vi "GetStatus.vi"(8 "error in (no error)":errorcluster, 11 "S4ACS_GUI in":refnum<class "S4GUI.lvclass">) -> (0 "error out":errorcluster, 1 "output cluster":T2={"Trigger Mode Status"="", "String output"="", "Instrument Status"={"WPROT pos"=0.0, "WPSEL pos"=0.0, "GMIR pos"=0.0, "GFOC pos"=0.0, "CALW pos"=0.0, "ASEL pos"=0.0, "connection"=FALSE}, "Sync Box State"=0, "Trigger General Status"="", "Instrument States"={"WPSEL State"=0, "WPROT State"=0, "CALW State"=0, "ASEL State"=0, "GMIR State"=0, "GFOC State"=0}, "Instrument Pos Names"={"WPROT posname"="", "WPSEL posname"="", "CALW posname"="", "ASEL posname"=""}, "ChannelA_Status"={"Current exp"=0.0, "Frames done"=0, "LastFileImage"="", "CamStatus"="", "Run state"=0, "connection"=FALSE, "Cooler ON/OFF"=0, "Currently temperature"=20, "Temperature Status"=""}, "WPROT seq"=0, "ChannelB_Status"={"Current exp"=0.0, "Frames done"=0, "LastFileImage"="", "CamStatus"="", "Run state"=0, "connection"=FALSE, "Cooler ON/OFF"=0, "Currently temperature"=20, "Temperature Status"=""}, "ChannelC_Status"={"Current exp"=0.0, "Frames done"=0, "LastFileImage"="", "CamStatus"="", "Run state"=0, "connection"=FALSE, "Cooler ON/OFF"=0, "Currently temperature"=20, "Temperature Status"=""}, "ChannelD_Status"={"Current exp"=0.0, "Frames done"=0, "LastFileImage"="", "CamStatus"="", "Run state"=0, "connection"=FALSE, "Cooler ON/OFF"=0, "Currently temperature"=20, "Temperature Status"=""}, "ChannelA_CCD"={"ACQUISITION_MODE"=1, "TRIGGER_MODE"=0, "READ_MODE"=4, "PREAMP"=0, "READOUT_RATE"=0, "VERTICAL_SHIFT_SPEED"=3, "EM_MODE"=0, "EM_GAIN"=2, "SHUTTER_MODE"=2, "SHUTTER_TTL"=0, "SHUTTER_OPENNING_TIME"=50, "SHUTTER_CLOSING_TIME"=50, "VBIN"=1, "HBIN"=1, "INITIAL_LINE"=1, "INITIAL_COLUMN"=1, "FINAL_LINE"=1024, "FINAL_COLUMN"=1024, "FRAME_TRANSFER"=FALSE, "VERTICAL_CLOCK_VOLTAGE"=0, "AD_CHANNEL"=0}, "ChannelB_CCD "={"ACQUISITION_MODE"=1, "TRIGGER_MODE"=0, "READ_MODE"=4, "PREAMP"=0, "READOUT_RATE"=0, "VERTICAL_SHIFT_SPEED"=3, "EM_MODE"=0, "EM_GAIN"=2, "SHUTTER_MODE"=2, "SHUTTER_TTL"=0, "SHUTTER_OPENNING_TIME"=50, "SHUTTER_CLOSING_TIME"=50, "VBIN"=1, "HBIN"=1, "INITIAL_LINE"=1, "INITIAL_COLUMN"=1, "FINAL_LINE"=1024, "FINAL_COLUMN"=1024, "FRAME_TRANSFER"=FALSE, "VERTICAL_CLOCK_VOLTAGE"=0, "AD_CHANNEL"=0}, "ChannelC_CCD"={"ACQUISITION_MODE"=1, "TRIGGER_MODE"=0, "READ_MODE"=4, "PREAMP"=0, "READOUT_RATE"=0, "VERTICAL_SHIFT_SPEED"=3, "EM_MODE"=0, "EM_GAIN"=2, "SHUTTER_MODE"=2, "SHUTTER_TTL"=0, "SHUTTER_OPENNING_TIME"=50, "SHUTTER_CLOSING_TIME"=50, "VBIN"=1, "HBIN"=1, "INITIAL_LINE"=1, "INITIAL_COLUMN"=1, "FINAL_LINE"=1024, "FINAL_COLUMN"=1024, "FRAME_TRANSFER"=FALSE, "VERTICAL_CLOCK_VOLTAGE"=0, "AD_CHANNEL"=0}, "ChannelD_CCD"={"ACQUISITION_MODE"=1, "TRIGGER_MODE"=0, "READ_MODE"=4, "PREAMP"=0, "READOUT_RATE"=0, "VERTICAL_SHIFT_SPEED"=3, "EM_MODE"=0, "EM_GAIN"=2, "SHUTTER_MODE"=2, "SHUTTER_TTL"=0, "SHUTTER_OPENNING_TIME"=50, "SHUTTER_CLOSING_TIME"=50, "VBIN"=1, "HBIN"=1, "INITIAL_LINE"=1, "INITIAL_COLUMN"=1, "FINAL_LINE"=1024, "FINAL_COLUMN"=1024, "FRAME_TRANSFER"=FALSE, "VERTICAL_CLOCK_VOLTAGE"=0, "AD_CHANNEL"=0}, "CHA_Checked Params"={"ACQUISITION_MODE"=FALSE, "TRIGGER_MODE"=FALSE, "READ_MODE"=FALSE, "PREAMP"=FALSE, "READOUT_RATE"=FALSE, "VERTICAL_SHIFT_SPEED"=FALSE, "EM_MODE"=FALSE, "EM_GAIN"=FALSE, "SHUTTER_MODE"=FALSE, "SHUTTER_TTL"=FALSE, "SHUTTER_OPENING_TIME"=FALSE, "SHUTTER_CLOSING_TIME"=FALSE, "VBIN"=FALSE, "HBIN"=FALSE, "INITIAL_LINE"=FALSE, "INITIAL_COLUMN"=FALSE, "FINAL_LINE"=FALSE, "FINAL_COLUMN"=FALSE, "FRAME_TRANSFER"=FALSE, "VERTICAL_CLOCK_VOLTAGE"=FALSE, "AD_CHANNEL"=FALSE}, "CHB_Checked Params"={"ACQUISITION_MODE"=FALSE, "TRIGGER_MODE"=FALSE, "READ_MODE"=FALSE, "PREAMP"=FALSE, "READOUT_RATE"=FALSE, "VERTICAL_SHIFT_SPEED"=FALSE, "EM_MODE"=FALSE, "EM_GAIN"=FALSE, "SHUTTER_MODE"=FALSE, "SHUTTER_TTL"=FALSE, "SHUTTER_OPENING_TIME"=FALSE, "SHUTTER_CLOSING_TIME"=FALSE, "VBIN"=FALSE, "HBIN"=FALSE, "INITIAL_LINE"=FALSE, "INITIAL_COLUMN"=FALSE, "FINAL_LINE"=FALSE, "FINAL_COLUMN"=FALSE, "FRAME_TRANSFER"=FALSE, "VERTICAL_CLOCK_VOLTAGE"=FALSE, "AD_CHANNEL"=FALSE}, "CHC_Checked Params"={"ACQUISITION_MODE"=FALSE, "TRIGGER_MODE"=FALSE, "READ_MODE"=FALSE, "PREAMP"=FALSE, "READOUT_RATE"=FALSE, "VERTICAL_SHIFT_SPEED"=FALSE, "EM_MODE"=FALSE, "EM_GAIN"=FALSE, "SHUTTER_MODE"=FALSE, "SHUTTER_TTL"=FALSE, "SHUTTER_OPENING_TIME"=FALSE, "SHUTTER_CLOSING_TIME"=FALSE, "VBIN"=FALSE, "HBIN"=FALSE, "INITIAL_LINE"=FALSE, "INITIAL_COLUMN"=FALSE, "FINAL_LINE"=FALSE, "FINAL_COLUMN"=FALSE, "FRAME_TRANSFER"=FALSE, "VERTICAL_CLOCK_VOLTAGE"=FALSE, "AD_CHANNEL"=FALSE}, "CHD_Checked Params"={"ACQUISITION_MODE"=FALSE, "TRIGGER_MODE"=FALSE, "READ_MODE"=FALSE, "PREAMP"=FALSE, "READOUT_RATE"=FALSE, "VERTICAL_SHIFT_SPEED"=FALSE, "EM_MODE"=FALSE, "EM_GAIN"=FALSE, "SHUTTER_MODE"=FALSE, "SHUTTER_TTL"=FALSE, "SHUTTER_OPENING_TIME"=FALSE, "SHUTTER_CLOSING_TIME"=FALSE, "VBIN"=FALSE, "HBIN"=FALSE, "INITIAL_LINE"=FALSE, "INITIAL_COLUMN"=FALSE, "FINAL_LINE"=FALSE, "FINAL_COLUMN"=FALSE, "FRAME_TRANSFER"=FALSE, "VERTICAL_CLOCK_VOLTAGE"=FALSE, "AD_CHANNEL"=FALSE}, "Trigger_connection"=FALSE, "TCSPD_connection"=FALSE} {"ChannelD_CCD"."VERTICAL_CLOCK_VOLTAGE" items=["Normal", "+1", "+2", "+3", "+4"]; "ChannelD_CCD"."SHUTTER_TTL" items=["TTL Low", "TTl High"]; "ChannelD_CCD"."SHUTTER_MODE" items=["Fully Auto", "OPEN", "CLOSED"]; "ChannelD_CCD"."EM_MODE" items=["Electron Multiplying", "Conventional"]; "ChannelD_CCD"."VERTICAL_SHIFT_SPEED" items=["0.6", "1.13", "2.2", "4.33"]; "ChannelD_CCD"."READOUT_RATE" items=["1 MHz", "0.1 MHz", "10 MHz", "20 MHz", "30 MHz"]; "ChannelD_CCD"."PREAMP" items=["Gain 1", "Gain 2"]; "ChannelD_CCD"."READ_MODE" items=["Full Vertical Binning", "Multi-Track", "Random-track", "Single-Track", "Image"]; "ChannelD_CCD"."TRIGGER_MODE" items=["Internal", "External", "N/A", "N/A", "N/A", "N/A", "External Start"]; "ChannelD_CCD"."ACQUISITION_MODE" items=["None", "Single", "Accumulate", "Kinetics", "Fast Kinetics"]; "ChannelC_CCD"."VERTICAL_CLOCK_VOLTAGE" items=["Normal", "+1", "+2", "+3", "+4"]; "ChannelC_CCD"."SHUTTER_TTL" items=["TTL Low", "TTl High"]; "ChannelC_CCD"."SHUTTER_MODE" items=["Fully Auto", "OPEN", "CLOSED"]; "ChannelC_CCD"."EM_MODE" items=["Electron Multiplying", "Conventional"]; "ChannelC_CCD"."VERTICAL_SHIFT_SPEED" items=["0.6", "1.13", "2.2", "4.33"]; "ChannelC_CCD"."READOUT_RATE" items=["1 MHz", "0 .1 MHz", "10 MHz", "20 MHz", "30 MHz"]; "ChannelC_CCD"."PREAMP" items=["Gain 1", "Gain 2"]; "ChannelC_CCD"."READ_MODE" items=["Full Vertical Binning", "Multi-Track", "Random-track", "Single-Track", "Image"]; "ChannelC_CCD"."TRIGGER_MODE" items=["Internal", "External", "N/A", "N/A", "N/A", "N/A", "External Start"]; "ChannelC_CCD"."ACQUISITION_MODE" items=["None", "Single", "Accumulate", "Kinetics", "Fast Kinetics"]; "ChannelB_CCD"."VERTICAL_CLOCK_VOLTAGE" items=["Normal", "+1", "+2", "+3", "+4"]; "ChannelB_CCD"."SHUTTER_TTL" items=["TTL Low", "TTl High"]; "ChannelB_CCD"."SHUTTER_MODE" items=["Fully Auto", "OPEN", "CLOSED"]; "ChannelB_CCD"."EM_MODE" items=["Electron Multiplying", "Conventional"]; "ChannelB_CCD"."VERTICAL_SHIFT_SPEED" items=["0.6", "1.13", "2.2", "4.33"]; "ChannelB_CCD"."READOUT_RATE" items=["1 MHz", "0.1 MHz", "10 MHz", "20 MHz", "30 MHz"]; "ChannelB_CCD"."PREAMP" items=["Gain 1", "Gain 2"]; "ChannelB_CCD"."READ_MODE" items=["Full Vertical Binning", "Multi-Track", "Random-track", "Single-Track", "Image"]; "ChannelB_CCD"."TRIGGER_MODE" items=["Internal", "External", "N/A", "N/A", "N/A", "N/A", "External Start"]; "ChannelB_CCD"."ACQUISITION_MODE" items=["None", "Single", "Accumulate", "Kinetics", "Fast Kinetics"]; "ChannelA_CCD"."VERTICAL_CLOCK_VOLTAGE" items=["Normal", "+1", "+2", "+3", "+4"]; "ChannelA_CCD"."SHUTTER_TTL" items=["TTL Low", "TTl High"]; "ChannelA_CCD"."SHUTTER_MODE" items=["Fully Auto", "OPEN", "CLOSED"]; "ChannelA_CCD"."EM_MODE" items=["Electron Multiplying", "Conventional"]; "ChannelA_CCD"."VERTICAL_SHIFT_SPEED" items=["0.6", "1.13", "2.2", "4.33"]; "ChannelA_CCD"."READOUT_RATE" items=["1 MHz", "0.1 MHz", "10 MHz", "20 MHz", "30 MHz"]; "ChannelA_CCD"."PREAMP" items=["Gain 1", "Gain 2"]; "ChannelA_CCD"."READ_MODE" items=["Full Vertical Binning", "Multi-Track", "Random-track", "Single-Track", "Image"]; "ChannelA_CCD"."TRIGGER_MODE" items=["Internal", "External", "N/A", "N/A", "N/A", "N/A", "External Start"]; "ChannelA_CCD"."ACQUISITION_MODE" items=["None", "Single", "Accumulate", "Kinetics", "Fast Kinetics"]; "ChannelD_Status"."Currently temperature" min=0 max=0; "ChannelD_Status"."Cooler ON/OFF" items=["Cooler OFF", "Cooler ON"]; "ChannelC_Status"."Currently temperature" min=0 max=0; "ChannelC_Status"."Cooler ON/OFF" items=["Cooler OFF", "Cooler ON"]; "ChannelB_Status"."Currently temperature" min=0 max=0; "ChannelB_Status"."Cooler ON/OFF" items=["Cooler OFF", "Cooler ON"]; "ChannelA_Status"."Currently temperature" min=0 max=0; "ChannelA_Status"."Cooler ON/OFF" items=["Cooler OFF", "Cooler ON"]}, 2 "Cluster Disable":T1, 3 "S4ACS_GUI out":refnum<class "S4GUI.lvclass">)   [LabVIEW 2018, in "S4GUI.lvclass"]
uses:
  S4GUI.lvclass
  S4GUI.lvclass/S4GUI.ctl
  Server/Server.lvclass/Server.ctl
  Instrument/Instrument.lvclass/Instrument.ctl
  Device/Optics/Optics.lvclass/Optics.ctl
  Interface/Interface.lvclass/Interface.ctl
  TCS/TCS.lvclass
  C:/Users/observer/Desktop/Sparc4GUI/SPARC4_GUI/Server/Server.lvclass
  SyncBox/Sync Box.lvclass
  Device/Optics/Opt_Selector/Opt_Selector.lvclass
  C:/Users/observer/Desktop/Sparc4GUI/SPARC4_GUI/Device/Optics/Optics.lvclass
  Device/Optics/Opt_Continuous/Opt_Continuous.lvclass
  Instrument/Instrument.lvclass
  Acquisition/Acquisition.lvclass
  Channel/Channel.lvclass
  Interface/Interface.lvclass
  Trigger/Trigger.lvclass
  Device/Optics/Optics.lvclass
  Server/Server.lvclass
panel:
  in  "Cluster":T3={"Trigger Mode Status"="", "String output"="", "Instrument Status"={"WPROT pos"=0.0, "WPSEL pos"=0.0, "GMIR pos"=0.0, "GFOC pos"=0.0, "CALW pos"=0.0, "ASEL pos"=0.0, "connection"=FALSE}, "Sync Box State"=0, "Trigger General Status"="", "Instrument States"={"WPSEL State"=0, "WPROT State"=0, "CALW State"=0, "ASEL State"=0, "GMIR State"=0, "GFOC State"=0}, "Instrument Pos Names"={"WPROT posname"="", "WPSEL posname"="", "CALW posname"="", "ASEL posname"=""}, "ChannelA_Status"={"Current exp"=0.0, "Frames done"=0, "LastFileImage"="", "CamStatus"="", "Run state"=0, "connection"=FALSE, "Cooler ON/OFF"=0, "Currently temperature"=20, "Temperature Status"=""}, "WPROT seq"=0, "ChannelB_Status"={"Current exp"=0.0, "Frames done"=0, "LastFileImage"="", "CamStatus"="", "Run state"=0, "connection"=FALSE, "Cooler ON/OFF"=0, "Currently temperature"=20, "Temperature Status"=""}, "ChannelC_Status"={"Current exp"=0.0, "Frames done"=0, "LastFileImage"="", "CamStatus"="", "Run state"=0, "connection"=FALSE, "Cooler ON/OFF"=0, "Currently temperature"=20, "Temperature Status"=""}, "ChannelD_Status"={"Current exp"=0.0, "Frames done"=0, "LastFileImage"="", "CamStatus"="", "Run state"=0, "connection"=FALSE, "Cooler ON/OFF"=0, "Currently temperature"=20, "Temperature Status"=""}, "ChannelA_CCD"={"ACQUISITION_MODE"=1, "TRIGGER_MODE"=0, "READ_MODE"=4, "PREAMP"=0, "READOUT_RATE"=0, "VERTICAL_SHIFT_SPEED"=3, "EM_MODE"=0, "EM_GAIN"=2, "SHUTTER_MODE"=2, "SHUTTER_TTL"=0, "SHUTTER_OPENNING_TIME"=50, "SHUTTER_CLOSING_TIME"=50, "VBIN"=1, "HBIN"=1, "INITIAL_LINE"=1, "INITIAL_COLUMN"=1, "FINAL_LINE"=1024, "FINAL_COLUMN"=1024, "FRAME_TRANSFER"=FALSE, "VERTICAL_CLOCK_VOLTAGE"=0, "AD_CHANNEL"=0}, "ChannelB_CCD"={"ACQUISITION_MODE"=1, "TRIGGER_MODE"=0, "READ_MODE"=4, "PREAMP"=0, "READOUT_RATE"=0, "VERTICAL_SHIFT_SPEED"=3, "EM_MODE"=0, "EM_GAIN"=2, "SHUTTER_MODE"=2, "SHUTTER_TTL"=0, "SHUTTER_OPENNING_TIME"=50, "SHUTTER_CLOSING_TIME"=50, "VBIN"=1, "HBIN"=1, "INITIAL_LINE"=1, "INITIAL_COLUMN"=1, "FINAL_LINE"=1024, "FINAL_COLUMN"=1024, "FRAME_TRANSFER"=FALSE, "VERTICAL_CLOCK_VOLTAGE"=0, "AD_CHANNEL"=0}, "ChannelC_CCD"={"ACQUISITION_MODE"=1, "TRIGGER_MODE"=0, "READ_MODE"=4, "PREAMP"=0, "READOUT_RATE"=0, "VERTICAL_SHIFT_SPEED"=3, "EM_MODE"=0, "EM_GAIN"=2, "SHUTTER_MODE"=2, "SHUTTER_TTL"=0, "SHUTTER_OPENNING_TIME"=50, "SHUTTER_CLOSING_TIME"=50, "VBIN"=1, "HBIN"=1, "INITIAL_LINE"=1, "INITIAL_COLUMN"=1, "FINAL_LINE"=1024, "FINAL_COLUMN"=1024, "FRAME_TRANSFER"=FALSE, "VERTICAL_CLOCK_VOLTAGE"=0, "AD_CHANNEL"=0}, "ChannelD_CCD"={"ACQUISITION_MODE"=1, "TRIGGER_MODE"=0, "READ_MODE"=4, "PREAMP"=0, "READOUT_RATE"=0, "VERTICAL_SHIFT_SPEED"=3, "EM_MODE"=0, "EM_GAIN"=2, "SHUTTER_MODE"=2, "SHUTTER_TTL"=0, "SHUTTER_OPENNING_TIME"=50, "SHUTTER_CLOSING_TIME"=50, "VBIN"=1, "HBIN"=1, "INITIAL_LINE"=1, "INITIAL_COLUMN"=1, "FINAL_LINE"=1024, "FINAL_COLUMN"=1024, "FRAME_TRANSFER"=FALSE, "VERTICAL_CLOCK_VOLTAGE"=0, "AD_CHANNEL"=0}, "CHA_Checked Params"={"ACQUISITION_MODE"=FALSE, "TRIGGER_MODE"=FALSE, "READ_MODE"=FALSE, "PREAMP"=FALSE, "READOUT_RATE"=FALSE, "VERTICAL_SHIFT_SPEED"=FALSE, "EM_MODE"=FALSE, "EM_GAIN"=FALSE, "SHUTTER_MODE"=FALSE, "SHUTTER_TTL"=FALSE, "SHUTTER_OPENING_TIME"=FALSE, "SHUTTER_CLOSING_TIME"=FALSE, "VBIN"=FALSE, "HBIN"=FALSE, "INITIAL_LINE"=FALSE, "INITIAL_COLUMN"=FALSE, "FINAL_LINE"=FALSE, "FINAL_COLUMN"=FALSE, "FRAME_TRANSFER"=FALSE, "VERTICAL_CLOCK_VOLTAGE"=FALSE, "AD_CHANNEL"=FALSE}, "CHB_Checked Params"={"ACQUISITION_MODE"=FALSE, "TRIGGER_MODE"=FALSE, "READ_MODE"=FALSE, "PREAMP"=FALSE, "READOUT_RATE"=FALSE, "VERTICAL_SHIFT_SPEED"=FALSE, "EM_MODE"=FALSE, "EM_GAIN"=FALSE, "SHUTTER_MODE"=FALSE, "SHUTTER_TTL"=FALSE, "SHUTTER_OPENING_TIME"=FALSE, "SHUTTER_CLOSING_TIME"=FALSE, "VBIN"=FALSE, "HBIN"=FALSE, "INITIAL_LINE"=FALSE, "INITIAL_COLUMN"=FALSE, "FINAL_LINE"=FALSE, "FINAL_COLUMN"=FALSE, "FRAME_TRANSFER"=FALSE, "VERTICAL_CLOCK_VOLTAGE"=FALSE, "AD_CHANNEL"=FALSE}, "CHC_Checked Params"={"ACQUISITION_MODE"=FALSE, "TRIGGER_MODE"=FALSE, "READ_MODE"=FALSE, "PREAMP"=FALSE, "READOUT_RATE"=FALSE, "VERTICAL_SHIFT_SPEED"=FALSE, "EM_MODE"=FALSE, "EM_GAIN"=FALSE, "SHUTTER_MODE"=FALSE, "SHUTTER_TTL"=FALSE, "SHUTTER_OPENING_TIME"=FALSE, "SHUTTER_CLOSING_TIME"=FALSE, "VBIN"=FALSE, "HBIN"=FALSE, "INITIAL_LINE"=FALSE, "INITIAL_COLUMN"=FALSE, "FINAL_LINE"=FALSE, "FINAL_COLUMN"=FALSE, "FRAME_TRANSFER"=FALSE, "VERTICAL_CLOCK_VOLTAGE"=FALSE, "AD_CHANNEL"=FALSE}, "CHD_Checked Params"={"ACQUISITION_MODE"=FALSE, "TRIGGER_MODE"=FALSE, "READ_MODE"=FALSE, "PREAMP"=FALSE, "READOUT_RATE"=FALSE, "VERTICAL_SHIFT_SPEED"=FALSE, "EM_MODE"=FALSE, "EM_GAIN"=FALSE, "SHUTTER_MODE"=FALSE, "SHUTTER_TTL"=FALSE, "SHUTTER_OPENING_TIME"=FALSE, "SHUTTER_CLOSING_TIME"=FALSE, "VBIN"=FALSE, "HBIN"=FALSE, "INITIAL_LINE"=FALSE, "INITIAL_COLUMN"=FALSE, "FINAL_LINE"=FALSE, "FINAL_COLUMN"=FALSE, "FRAME_TRANSFER"=FALSE, "VERTICAL_CLOCK_VOLTAGE"=FALSE, "AD_CHANNEL"=FALSE}, "Trigger_connection"=FALSE, "TCSPD_connection"=FALSE} {"ChannelD_CCD"."VERTICAL_CLOCK_VOLTAGE" items=["Normal", "+1", "+2", "+3", "+4"]; "ChannelD_CCD"."SHUTTER_TTL" items=["TTL Low", "TTl High"]; "ChannelD_CCD"."SHUTTER_MODE" items=["Fully Auto", "OPEN", "CLOSED"]; "ChannelD_CCD"."EM_MODE" items=["Electron Multiplying", "Conventional"]; "ChannelD_CCD"."VERTICAL_SHIFT_SPEED" items=["0.6", "1.13", "2.2", "4.33"]; "ChannelD_CCD"."READOUT_RATE" items=["1 MHz", "0.1 MHz", "10 MHz", "20 MHz", "30 MHz"]; "ChannelD_CCD"."PREAMP" items=["Gain 1", "Gain 2"]; "ChannelD_CCD"."READ_MODE" items=["Full Vertical Binning", "Multi-Track", "Random-track", "Single-Track", "Image"]; "ChannelD_CCD"."TRIGGER_MODE" items=["Internal", "External", "N/A", "N/A", "N/A", "N/A", "External Start"]; "ChannelD_CCD"."ACQUISITION_MODE" items=["None", "Single", "Accumulate", "Kinetics", "Fast Kinetics"]; "ChannelC_CCD"."VERTICAL_CLOCK_VOLTAGE" items=["Normal", "+1", "+2", "+3", "+4"]; "ChannelC_CCD"."SHUTTER_TTL" items=["TTL Low", "TTl High"]; "ChannelC_CCD"."SHUTTER_MODE" items=["Fully Auto", "OPEN", "CLOSED"]; "ChannelC_CCD"."EM_MODE" items=["Electron Multiplying", "Conventional"]; "ChannelC_CCD"."VERTICAL_SHIFT_SPEED" items=["0.6", "1.13", "2.2", "4.33"]; "ChannelC_CCD"."READOUT_RATE" items=["1 MHz", "0.1 MHz", "10 MHz", "20 MHz", "30 MHz"]; "ChannelC_CCD"."PREAMP" items=["Gain 1", "Gain 2"]; "ChannelC_CCD"."READ_MODE" items=["Full Vertical Binning", "Multi-Track", "Random-track", "Single-Track", "Image"]; "ChannelC_CCD"."TRIGGER_MODE" items=["Internal", "External", "N/A", "N/A", "N/A", "N/A", "External Start"]; "ChannelC_CCD"."ACQUISITION_MODE" items=["None", "Single", "Accumulate", "Kinetics", "Fast Kinetics"]; "ChannelB_CCD"."VERTICAL_CLOCK_VOLTAGE" items=["Normal", "+1", "+2", "+3", "+4"]; "ChannelB_CCD"."SHUTTER_TTL" items=["TTL Low", "TTl High"]; "ChannelB_CCD"."SHUTTER_MODE" items=["Fully Auto", "OPEN", "CLOSED"]; "ChannelB_CCD"."EM_MODE" items=["Electron Multiplying", "Conventional"]; "ChannelB_CCD"."VERTICAL_SHIFT_SPEED" items=["0.6", "1.13", "2.2", "4.33"]; "ChannelB_CCD"."READOUT_RATE" items=["1 MHz", "0.1 MHz", "10 MHz", "20 MHz", "30 MHz"]; "ChannelB_CCD"."PREAMP" items=["Gain 1", "Gain 2"]; "ChannelB_CCD"."READ_MODE" items=["Full Vertical Binning", "Multi-Track", "Random-track", "Single-Track", "Image"]; "ChannelB_CCD"."TRIGGER_MODE" items=["Internal", "External", "N/A", "N/A", "N/A", "N/A", "External Start"]; "ChannelB_CCD"."ACQUISITION_MODE" items=["None", "Single", "Accumulate", "Kinetics", "Fast Kinetics"]; "ChannelA_CCD"."VERTICAL_CLOCK_VOLTAGE" items=["Normal", "+1", "+2", "+3", "+4"]; "ChannelA_CCD"."SHUTTER_TTL" items=["TTL Low", "TTl High"]; "ChannelA_CCD"."SHUTTER_MODE" items=["Fully Auto", "OPEN", "CLOSED"]; "ChannelA_CCD"."EM_MODE" items=["Electron Multiplying", "Conventional"]; "ChannelA_CCD"."VERTICAL_SHIFT_SPEED" items=["0.6", "1.13", "2.2", "4.33"]; "ChannelA_CCD"."READOUT_RATE" items=["1 MHz", "0.1 MHz", "10 MHz", "20 MHz", "30 MHz"]; "ChannelA_CCD"."PREAMP" items=["Gain 1", "Gain 2"]; "ChannelA_CCD"."READ_MODE" items=["Full Vertical Binning", "Multi-Track", "Random-track", "Single-Track", "Image"]; "ChannelA_CCD"."TRIGGER_MODE" items=["Internal", "External", "N/A", "N/A", "N/A", "N/A", "External Start"]; "ChannelA_CCD"."ACQUISITION_MODE" items=["None", "Single", "Accumulate", "Kinetics", "Fast Kinetics"]; "ChannelD_Status"."Currently temperature" min=0 max=0; "ChannelD_Status"."Cooler ON/OFF" items=["Cooler OFF", "Cooler ON"]; "ChannelC_Status"."Currently temperature" min=0 max=0; "ChannelC_Status"."Cooler ON/OFF" items=["Cooler OFF", "Cooler ON"]; "ChannelB_Status"."Currently temperature" min=0 max=0; "ChannelB_Status"."Cooler ON/OFF" items=["Cooler OFF", "Cooler ON"]; "ChannelA_Status"."Currently temperature" min=0 max=0; "ChannelA_Status"."Cooler ON/OFF" items=["Cooler OFF", "Cooler ON"]}
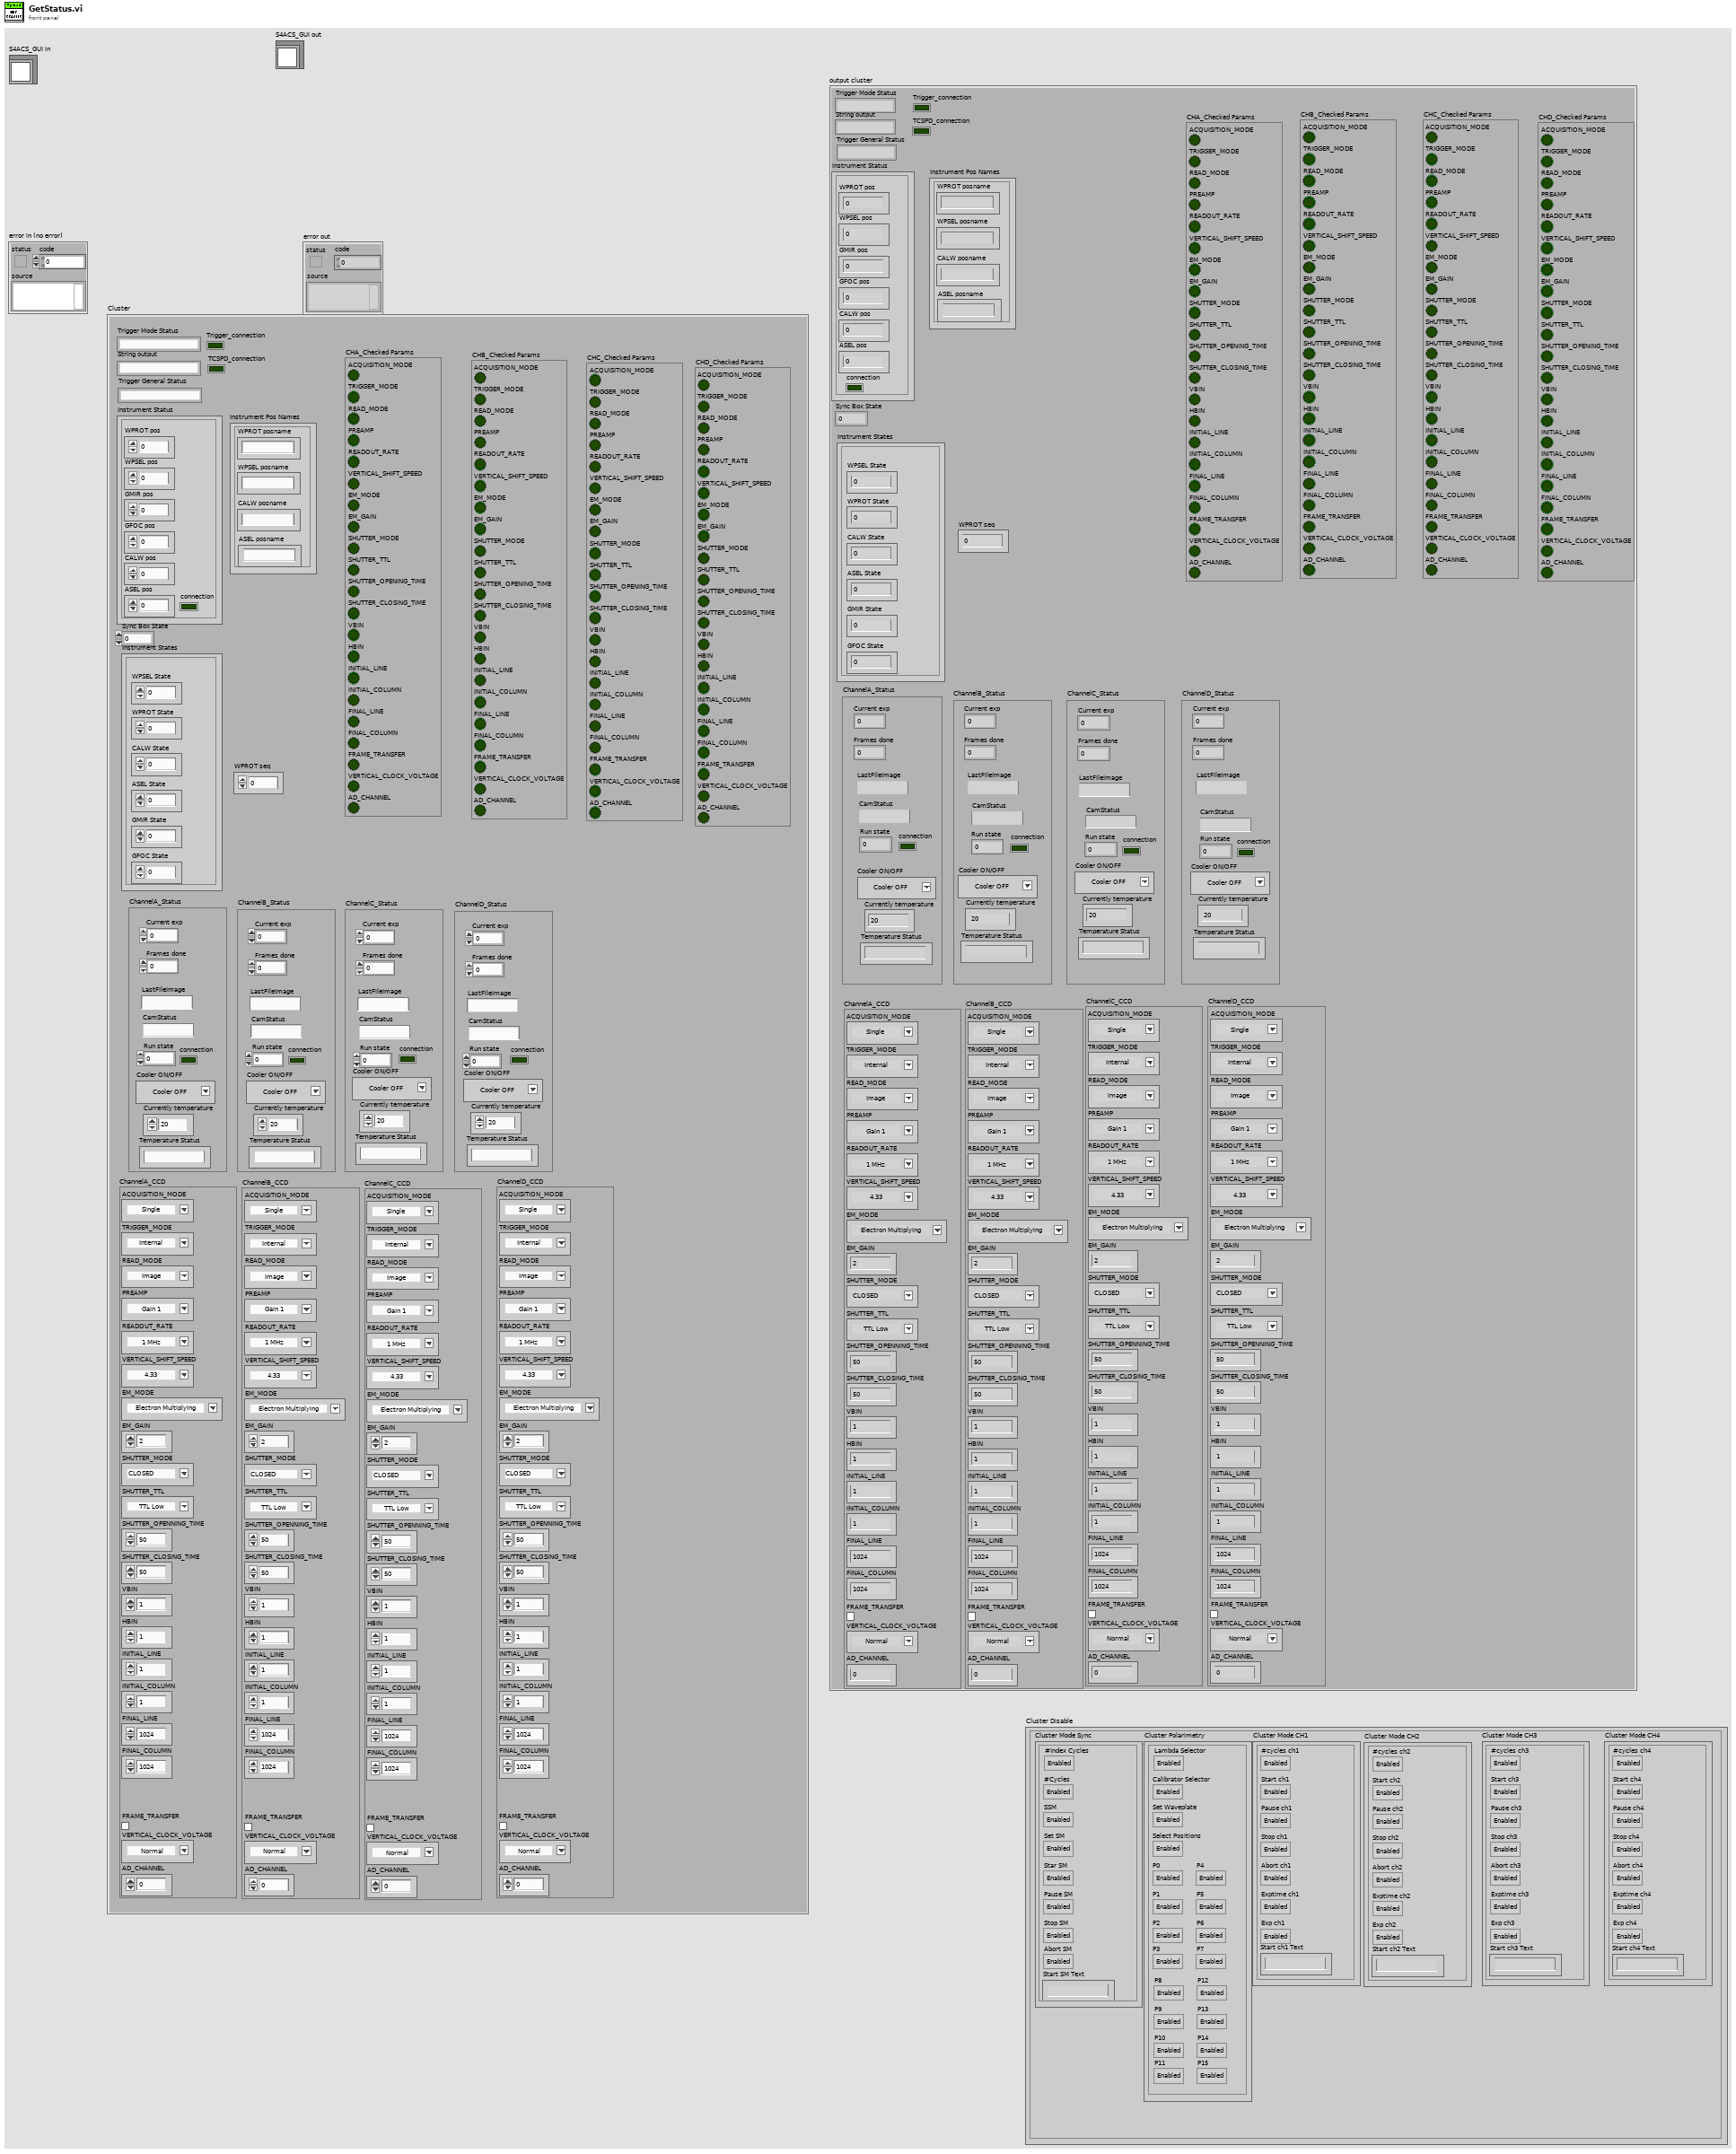
[diagram p1: front panel]
types:
  T1 = cluster{"Cluster Mode Sync":cluster{"#Index Cycles":enum8{"Enabled", "Disabled", "Disabled and Grayed Out"}, "#Cycles":enum8{"Enabled", "Disabled", "Disabled and Grayed Out"}, "SSM":enum8{"Enabled", "Disabled", "Disabled and Grayed Out"}, "Set SM":enum8{"Enabled", "Disabled", "Disabled and Grayed Out"}, "Star SM":enum8{"Enabled", "Disabled", "Disabled and Grayed Out"}, "Pause SM":enum8{"Enabled", "Disabled", "Disabled and Grayed Out"}, "Stop SM":enum8{"Enabled", "Disabled", "Disabled and Grayed Out"}, "Abort SM":enum8{"Enabled", "Disabled", "Disabled and Grayed Out"}, "Start SM Text":string}, "Cluster Polarimetry":cluster{"Lambda Selector":enum8{"Enabled", "Disabled", "Disabled and Grayed Out"}, "Calibrator Selector":enum8{"Enabled", "Disabled", "Disabled and Grayed Out"}, "Set Waveplate":enum8{"Enabled", "Disabled", "Disabled and Grayed Out"}, "Select Positions":enum8{"Enabled", "Disabled", "Disabled and Grayed Out"}, "P0":enum8{"Enabled", "Disabled", "Disabled and Grayed Out"}, "P1":enum8{"Enabled", "Disabled", "Disabled and Grayed Out"}, "P2":enum8{"Enabled", "Disabled", "Disabled and Grayed Out"}, "P3":enum8{"Enabled", "Disabled", "Disabled and Grayed Out"}, "P4":enum8{"Enabled", "Disabled", "Disabled and Grayed Out"}, "P5":enum8{"Enabled", "Disabled", "Disabled and Grayed Out"}, "P6":enum8{"Enabled", "Disabled", "Disabled and Grayed Out"}, "P7":enum8{"Enabled", "Disabled", "Disabled and Grayed Out"}, "P8":enum8{"Enabled", "Disabled", "Disabled and Grayed Out"}, "P9":enum8{"Enabled", "Disabled", "Disabled and Grayed Out"}, "P10":enum8{"Enabled", "Disabled", "Disabled and Grayed Out"}, "P11":enum8{"Enabled", "Disabled", "Disabled and Grayed Out"}, "P12":enum8{"Enabled", "Disabled", "Disabled and Grayed Out"}, "P13":enum8{"Enabled", "Disabled", "Disabled and Grayed Out"}, "P14":enum8{"Enabled", "Disabled", "Disabled and Grayed Out"}, "P15":enum8{"Enabled", "Disabled", "Disabled and Grayed Out"}}, "Cluster Mode CH1":cluster{"#cycles ch1":enum8{"Enabled", "Disabled", "Disabled and Grayed Out"}, "Start ch1":enum8{"Enabled", "Disabled", "Disabled and Grayed Out"}, "Pause ch1":enum8{"Enabled", "Disabled", "Disabled and Grayed Out"}, "Stop ch1":enum8{"Enabled", "Disabled", "Disabled and Grayed Out"}, "Abort ch1":enum8{"Enabled", "Disabled", "Disabled and Grayed Out"}, "Exptime ch1":enum8{"Enabled", "Disabled", "Disabled and Grayed Out"}, "Exp ch1":enum8{"Enabled", "Disabled", "Disabled and Grayed Out"}, "Start ch1 Text":string}, "Cluster Mode CH2":cluster{"#cycles ch2":enum8{"Enabled", "Disabled", "Disabled and Grayed Out"}, "Start ch2":enum8{"Enabled", "Disabled", "Disabled and Grayed Out"}, "Pause ch2":enum8{"Enabled", "Disabled", "Disabled and Grayed Out"}, "Stop ch2":enum8{"Enabled", "Disabled", "Disabled and Grayed Out"}, "Abort ch2":enum8{"Enabled", "Disabled", "Disabled and Grayed Out"}, "Exptime ch2":enum8{"Enabled", "Disabled", "Disabled and Grayed Out"}, "Exp ch2":enum8{"Enabled", "Disabled", "Disabled and Grayed Out"}, "Start ch2 Text":string}, "Cluster Mode CH3":cluster{"#cycles ch3":enum8{"Enabled", "Disabled", "Disabled and Grayed Out"}, "Start ch3":enum8{"Enabled", "Disabled", "Disabled and Grayed Out"}, "Pause ch3":enum8{"Enabled", "Disabled", "Disabled and Grayed Out"}, "Stop ch3":enum8{"Enabled", "Disabled", "Disabled and Grayed Out"}, "Abort ch3":enum8{"Enabled", "Disabled", "Disabled and Grayed Out"}, "Exptime ch3":enum8{"Enabled", "Disabled", "Disabled and Grayed Out"}, "Exp ch3":enum8{"Enabled", "Disabled", "Disabled and Grayed Out"}, "Start ch3 Text":string}, "Cluster Mode CH4":cluster{"#cycles ch4":enum8{"Enabled", "Disabled", "Disabled and Grayed Out"}, "Start ch4":enum8{"Enabled", "Disabled", "Disabled and Grayed Out"}, "Pause ch4":enum8{"Enabled", "Disabled", "Disabled and Grayed Out"}, "Stop ch4":enum8{"Enabled", "Disabled", "Disabled and Grayed Out"}, "Abort ch4":enum8{"Enabled", "Disabled", "Disabled and Grayed Out"}, "Exptime ch4":enum8{"Enabled", "Disabled", "Disabled and Grayed Out"}, "Exp ch4":enum8{"Enabled", "Disabled", "Disabled and Grayed Out"}, "Start ch4 Text":string}}
  T2 = cluster{"Trigger Mode Status":string, "String output":string, "Instrument Status":cluster{"WPROT pos":dbl, "WPSEL pos":dbl, "GMIR pos":dbl, "GFOC pos":dbl, "CALW pos":dbl, "ASEL pos":dbl, "connection":bool}, "Sync Box State":i32, "Trigger General Status":string, "Instrument States":cluster{"WPSEL State":i32, "WPROT State":i32, "CALW State":i32, "ASEL State":i32, "GMIR State":i32, "GFOC State":i32}, "Instrument Pos Names":cluster{"WPROT posname":string, "WPSEL posname":string, "CALW posname":string, "ASEL posname":string}, "ChannelA_Status":cluster{"Current exp":dbl, "Frames done":u32, "LastFileImage":string, "CamStatus":string, "Run state":u32, "connection":bool, "Cooler ON/OFF":i16, "Currently temperature":i16, "Temperature Status":string}, "WPROT seq":u16, "ChannelB_Status":cluster{"Current exp":dbl, "Frames done":u32, "LastFileImage":string, "CamStatus":string, "Run state":u32, "connection":bool, "Cooler ON/OFF":i16, "Currently temperature":i16, "Temperature Status":string}, "ChannelC_Status":cluster{"Current exp":dbl, "Frames done":u32, "LastFileImage":string, "CamStatus":string, "Run state":u32, "connection":bool, "Cooler ON/OFF":i16, "Currently temperature":i16, "Temperature Status":string}, "ChannelD_Status":cluster{"Current exp":dbl, "Frames done":u32, "LastFileImage":string, "CamStatus":string, "Run state":u32, "connection":bool, "Cooler ON/OFF":i16, "Currently temperature":i16, "Temperature Status":string}, "ChannelA_CCD":cluster{"ACQUISITION_MODE":u8, "TRIGGER_MODE":u8, "READ_MODE":u8, "PREAMP":u8, "READOUT_RATE":u8, "VERTICAL_SHIFT_SPEED":u8, "EM_MODE":u8, "EM_GAIN":u16, "SHUTTER_MODE":u8, "SHUTTER_TTL":u8, "SHUTTER_OPENNING_TIME":u16, "SHUTTER_CLOSING_TIME":u16, "VBIN":u16, "HBIN":u16, "INITIAL_LINE":u16, "INITIAL_COLUMN":u16, "FINAL_LINE":u16, "FINAL_COLUMN":u16, "FRAME_TRANSFER":bool, "VERTICAL_CLOCK_VOLTAGE":u8, "AD_CHANNEL":u32}, "ChannelB_CCD ":cluster{"ACQUISITION_MODE":u8, "TRIGGER_MODE":u8, "READ_MODE":u8, "PREAMP":u8, "READOUT_RATE":u8, "VERTICAL_SHIFT_SPEED":u8, "EM_MODE":u8, "EM_GAIN":u16, "SHUTTER_MODE":u8, "SHUTTER_TTL":u8, "SHUTTER_OPENNING_TIME":u16, "SHUTTER_CLOSING_TIME":u16, "VBIN":u16, "HBIN":u16, "INITIAL_LINE":u16, "INITIAL_COLUMN":u16, "FINAL_LINE":u16, "FINAL_COLUMN":u16, "FRAME_TRANSFER":bool, "VERTICAL_CLOCK_VOLTAGE":u8, "AD_CHANNEL":u32}, "ChannelC_CCD":cluster{"ACQUISITION_MODE":u8, "TRIGGER_MODE":u8, "READ_MODE":u8, "PREAMP":u8, "READOUT_RATE":u8, "VERTICAL_SHIFT_SPEED":u8, "EM_MODE":u8, "EM_GAIN":u16, "SHUTTER_MODE":u8, "SHUTTER_TTL":u8, "SHUTTER_OPENNING_TIME":u16, "SHUTTER_CLOSING_TIME":u16, "VBIN":u16, "HBIN":u16, "INITIAL_LINE":u16, "INITIAL_COLUMN":u16, "FINAL_LINE":u16, "FINAL_COLUMN":u16, "FRAME_TRANSFER":bool, "VERTICAL_CLOCK_VOLTAGE":u8, "AD_CHANNEL":u32}, "ChannelD_CCD":cluster{"ACQUISITION_MODE":u8, "TRIGGER_MODE":u8, "READ_MODE":u8, "PREAMP":u8, "READOUT_RATE":u8, "VERTICAL_SHIFT_SPEED":u8, "EM_MODE":u8, "EM_GAIN":u16, "SHUTTER_MODE":u8, "SHUTTER_TTL":u8, "SHUTTER_OPENNING_TIME":u16, "SHUTTER_CLOSING_TIME":u16, "VBIN":u16, "HBIN":u16, "INITIAL_LINE":u16, "INITIAL_COLUMN":u16, "FINAL_LINE":u16, "FINAL_COLUMN":u16, "FRAME_TRANSFER":bool, "VERTICAL_CLOCK_VOLTAGE":u8, "AD_CHANNEL":u32}, "CHA_Checked Params":cluster{"ACQUISITION_MODE":bool, "TRIGGER_MODE":bool, "READ_MODE":bool, "PREAMP":bool, "READOUT_RATE":bool, "VERTICAL_SHIFT_SPEED":bool, "EM_MODE":bool, "EM_GAIN":bool, "SHUTTER_MODE":bool, "SHUTTER_TTL":bool, "SHUTTER_OPENING_TIME":bool, "SHUTTER_CLOSING_TIME":bool, "VBIN":bool, "HBIN":bool, "INITIAL_LINE":bool, "INITIAL_COLUMN":bool, "FINAL_LINE":bool, "FINAL_COLUMN":bool, "FRAME_TRANSFER":bool, "VERTICAL_CLOCK_VOLTAGE":bool, "AD_CHANNEL":bool}, "CHB_Checked Params":cluster{"ACQUISITION_MODE":bool, "TRIGGER_MODE":bool, "READ_MODE":bool, "PREAMP":bool, "READOUT_RATE":bool, "VERTICAL_SHIFT_SPEED":bool, "EM_MODE":bool, "EM_GAIN":bool, "SHUTTER_MODE":bool, "SHUTTER_TTL":bool, "SHUTTER_OPENING_TIME":bool, "SHUTTER_CLOSING_TIME":bool, "VBIN":bool, "HBIN":bool, "INITIAL_LINE":bool, "INITIAL_COLUMN":bool, "FINAL_LINE":bool, "FINAL_COLUMN":bool, "FRAME_TRANSFER":bool, "VERTICAL_CLOCK_VOLTAGE":bool, "AD_CHANNEL":bool}, "CHC_Checked Params":cluster{"ACQUISITION_MODE":bool, "TRIGGER_MODE":bool, "READ_MODE":bool, "PREAMP":bool, "READOUT_RATE":bool, "VERTICAL_SHIFT_SPEED":bool, "EM_MODE":bool, "EM_GAIN":bool, "SHUTTER_MODE":bool, "SHUTTER_TTL":bool, "SHUTTER_OPENING_TIME":bool, "SHUTTER_CLOSING_TIME":bool, "VBIN":bool, "HBIN":bool, "INITIAL_LINE":bool, "INITIAL_COLUMN":bool, "FINAL_LINE":bool, "FINAL_COLUMN":bool, "FRAME_TRANSFER":bool, "VERTICAL_CLOCK_VOLTAGE":bool, "AD_CHANNEL":bool}, "CHD_Checked Params":cluster{"ACQUISITION_MODE":bool, "TRIGGER_MODE":bool, "READ_MODE":bool, "PREAMP":bool, "READOUT_RATE":bool, "VERTICAL_SHIFT_SPEED":bool, "EM_MODE":bool, "EM_GAIN":bool, "SHUTTER_MODE":bool, "SHUTTER_TTL":bool, "SHUTTER_OPENING_TIME":bool, "SHUTTER_CLOSING_TIME":bool, "VBIN":bool, "HBIN":bool, "INITIAL_LINE":bool, "INITIAL_COLUMN":bool, "FINAL_LINE":bool, "FINAL_COLUMN":bool, "FRAME_TRANSFER":bool, "VERTICAL_CLOCK_VOLTAGE":bool, "AD_CHANNEL":bool}, "Trigger_connection":bool, "TCSPD_connection":bool}
  T3 = cluster{"Trigger Mode Status":string, "String output":string, "Instrument Status":cluster{"WPROT pos":dbl, "WPSEL pos":dbl, "GMIR pos":dbl, "GFOC pos":dbl, "CALW pos":dbl, "ASEL pos":dbl, "connection":bool}, "Sync Box State":i32, "Trigger General Status":string, "Instrument States":cluster{"WPSEL State":i32, "WPROT State":i32, "CALW State":i32, "ASEL State":i32, "GMIR State":i32, "GFOC State":i32}, "Instrument Pos Names":cluster{"WPROT posname":string, "WPSEL posname":string, "CALW posname":string, "ASEL posname":string}, "ChannelA_Status":cluster{"Current exp":dbl, "Frames done":u32, "LastFileImage":string, "CamStatus":string, "Run state":u32, "connection":bool, "Cooler ON/OFF":i16, "Currently temperature":i16, "Temperature Status":string}, "WPROT seq":u16, "ChannelB_Status":cluster{"Current exp":dbl, "Frames done":u32, "LastFileImage":string, "CamStatus":string, "Run state":u32, "connection":bool, "Cooler ON/OFF":i16, "Currently temperature":i16, "Temperature Status":string}, "ChannelC_Status":cluster{"Current exp":dbl, "Frames done":u32, "LastFileImage":string, "CamStatus":string, "Run state":u32, "connection":bool, "Cooler ON/OFF":i16, "Currently temperature":i16, "Temperature Status":string}, "ChannelD_Status":cluster{"Current exp":dbl, "Frames done":u32, "LastFileImage":string, "CamStatus":string, "Run state":u32, "connection":bool, "Cooler ON/OFF":i16, "Currently temperature":i16, "Temperature Status":string}, "ChannelA_CCD":cluster{"ACQUISITION_MODE":u8, "TRIGGER_MODE":u8, "READ_MODE":u8, "PREAMP":u8, "READOUT_RATE":u8, "VERTICAL_SHIFT_SPEED":u8, "EM_MODE":u8, "EM_GAIN":u16, "SHUTTER_MODE":u8, "SHUTTER_TTL":u8, "SHUTTER_OPENNING_TIME":u16, "SHUTTER_CLOSING_TIME":u16, "VBIN":u16, "HBIN":u16, "INITIAL_LINE":u16, "INITIAL_COLUMN":u16, "FINAL_LINE":u16, "FINAL_COLUMN":u16, "FRAME_TRANSFER":bool, "VERTICAL_CLOCK_VOLTAGE":u8, "AD_CHANNEL":u32}, "ChannelB_CCD":cluster{"ACQUISITION_MODE":u8, "TRIGGER_MODE":u8, "READ_MODE":u8, "PREAMP":u8, "READOUT_RATE":u8, "VERTICAL_SHIFT_SPEED":u8, "EM_MODE":u8, "EM_GAIN":u16, "SHUTTER_MODE":u8, "SHUTTER_TTL":u8, "SHUTTER_OPENNING_TIME":u16, "SHUTTER_CLOSING_TIME":u16, "VBIN":u16, "HBIN":u16, "INITIAL_LINE":u16, "INITIAL_COLUMN":u16, "FINAL_LINE":u16, "FINAL_COLUMN":u16, "FRAME_TRANSFER":bool, "VERTICAL_CLOCK_VOLTAGE":u8, "AD_CHANNEL":u32}, "ChannelC_CCD":cluster{"ACQUISITION_MODE":u8, "TRIGGER_MODE":u8, "READ_MODE":u8, "PREAMP":u8, "READOUT_RATE":u8, "VERTICAL_SHIFT_SPEED":u8, "EM_MODE":u8, "EM_GAIN":u16, "SHUTTER_MODE":u8, "SHUTTER_TTL":u8, "SHUTTER_OPENNING_TIME":u16, "SHUTTER_CLOSING_TIME":u16, "VBIN":u16, "HBIN":u16, "INITIAL_LINE":u16, "INITIAL_COLUMN":u16, "FINAL_LINE":u16, "FINAL_COLUMN":u16, "FRAME_TRANSFER":bool, "VERTICAL_CLOCK_VOLTAGE":u8, "AD_CHANNEL":u32}, "ChannelD_CCD":cluster{"ACQUISITION_MODE":u8, "TRIGGER_MODE":u8, "READ_MODE":u8, "PREAMP":u8, "READOUT_RATE":u8, "VERTICAL_SHIFT_SPEED":u8, "EM_MODE":u8, "EM_GAIN":u16, "SHUTTER_MODE":u8, "SHUTTER_TTL":u8, "SHUTTER_OPENNING_TIME":u16, "SHUTTER_CLOSING_TIME":u16, "VBIN":u16, "HBIN":u16, "INITIAL_LINE":u16, "INITIAL_COLUMN":u16, "FINAL_LINE":u16, "FINAL_COLUMN":u16, "FRAME_TRANSFER":bool, "VERTICAL_CLOCK_VOLTAGE":u8, "AD_CHANNEL":u32}, "CHA_Checked Params":cluster{"ACQUISITION_MODE":bool, "TRIGGER_MODE":bool, "READ_MODE":bool, "PREAMP":bool, "READOUT_RATE":bool, "VERTICAL_SHIFT_SPEED":bool, "EM_MODE":bool, "EM_GAIN":bool, "SHUTTER_MODE":bool, "SHUTTER_TTL":bool, "SHUTTER_OPENING_TIME":bool, "SHUTTER_CLOSING_TIME":bool, "VBIN":bool, "HBIN":bool, "INITIAL_LINE":bool, "INITIAL_COLUMN":bool, "FINAL_LINE":bool, "FINAL_COLUMN":bool, "FRAME_TRANSFER":bool, "VERTICAL_CLOCK_VOLTAGE":bool, "AD_CHANNEL":bool}, "CHB_Checked Params":cluster{"ACQUISITION_MODE":bool, "TRIGGER_MODE":bool, "READ_MODE":bool, "PREAMP":bool, "READOUT_RATE":bool, "VERTICAL_SHIFT_SPEED":bool, "EM_MODE":bool, "EM_GAIN":bool, "SHUTTER_MODE":bool, "SHUTTER_TTL":bool, "SHUTTER_OPENING_TIME":bool, "SHUTTER_CLOSING_TIME":bool, "VBIN":bool, "HBIN":bool, "INITIAL_LINE":bool, "INITIAL_COLUMN":bool, "FINAL_LINE":bool, "FINAL_COLUMN":bool, "FRAME_TRANSFER":bool, "VERTICAL_CLOCK_VOLTAGE":bool, "AD_CHANNEL":bool}, "CHC_Checked Params":cluster{"ACQUISITION_MODE":bool, "TRIGGER_MODE":bool, "READ_MODE":bool, "PREAMP":bool, "READOUT_RATE":bool, "VERTICAL_SHIFT_SPEED":bool, "EM_MODE":bool, "EM_GAIN":bool, "SHUTTER_MODE":bool, "SHUTTER_TTL":bool, "SHUTTER_OPENING_TIME":bool, "SHUTTER_CLOSING_TIME":bool, "VBIN":bool, "HBIN":bool, "INITIAL_LINE":bool, "INITIAL_COLUMN":bool, "FINAL_LINE":bool, "FINAL_COLUMN":bool, "FRAME_TRANSFER":bool, "VERTICAL_CLOCK_VOLTAGE":bool, "AD_CHANNEL":bool}, "CHD_Checked Params":cluster{"ACQUISITION_MODE":bool, "TRIGGER_MODE":bool, "READ_MODE":bool, "PREAMP":bool, "READOUT_RATE":bool, "VERTICAL_SHIFT_SPEED":bool, "EM_MODE":bool, "EM_GAIN":bool, "SHUTTER_MODE":bool, "SHUTTER_TTL":bool, "SHUTTER_OPENING_TIME":bool, "SHUTTER_CLOSING_TIME":bool, "VBIN":bool, "HBIN":bool, "INITIAL_LINE":bool, "INITIAL_COLUMN":bool, "FINAL_LINE":bool, "FINAL_COLUMN":bool, "FRAME_TRANSFER":bool, "VERTICAL_CLOCK_VOLTAGE":bool, "AD_CHANNEL":bool}, "Trigger_connection":bool, "TCSPD_connection":bool}
  T4 = cluster{"ACQUISITION_MODE":bool, "TRIGGER_MODE":bool, "READ_MODE":bool, "PREAMP":bool, "READOUT_RATE":bool, "VERTICAL_SHIFT_SPEED":bool, "EM_MODE":bool, "EM_GAIN":bool, "SHUTTER_MODE":bool, "SHUTTER_TTL":bool, "SHUTTER_OPENING_TIME":bool, "SHUTTER_CLOSING_TIME":bool, "VBIN":bool, "HBIN":bool, "INITIAL_LINE":bool, "INITIAL_COLUMN":bool, "FINAL_LINE":bool, "FINAL_COLUMN":bool, "FRAME_TRANSFER":bool, "VERTICAL_CLOCK_VOLTAGE":bool, "AD_CHANNEL":bool}
  T5 = cluster{"ACQUISITION_MODE":u8, "TRIGGER_MODE":u8, "READ_MODE":u8, "PREAMP":u8, "READOUT_RATE":u8, "VERTICAL_SHIFT_SPEED":u8, "EM_MODE":u8, "EM_GAIN":u16, "SHUTTER_MODE":u8, "SHUTTER_TTL":u8, "SHUTTER_OPENING_TIME":u16, "SHUTTER_CLOSING_TIME":u16, "VBIN":u16, "HBIN":u16, "INITIAL_LINE":u16, "INITIAL_COLUMN":u16, "FINAL_LINE":u16, "FINAL_COLUMN":u16, "FRAME_TRANSFER":bool, "VERTICAL_CLOCK_VOLTAGE":u8, "AD_CHANNEL":u32}
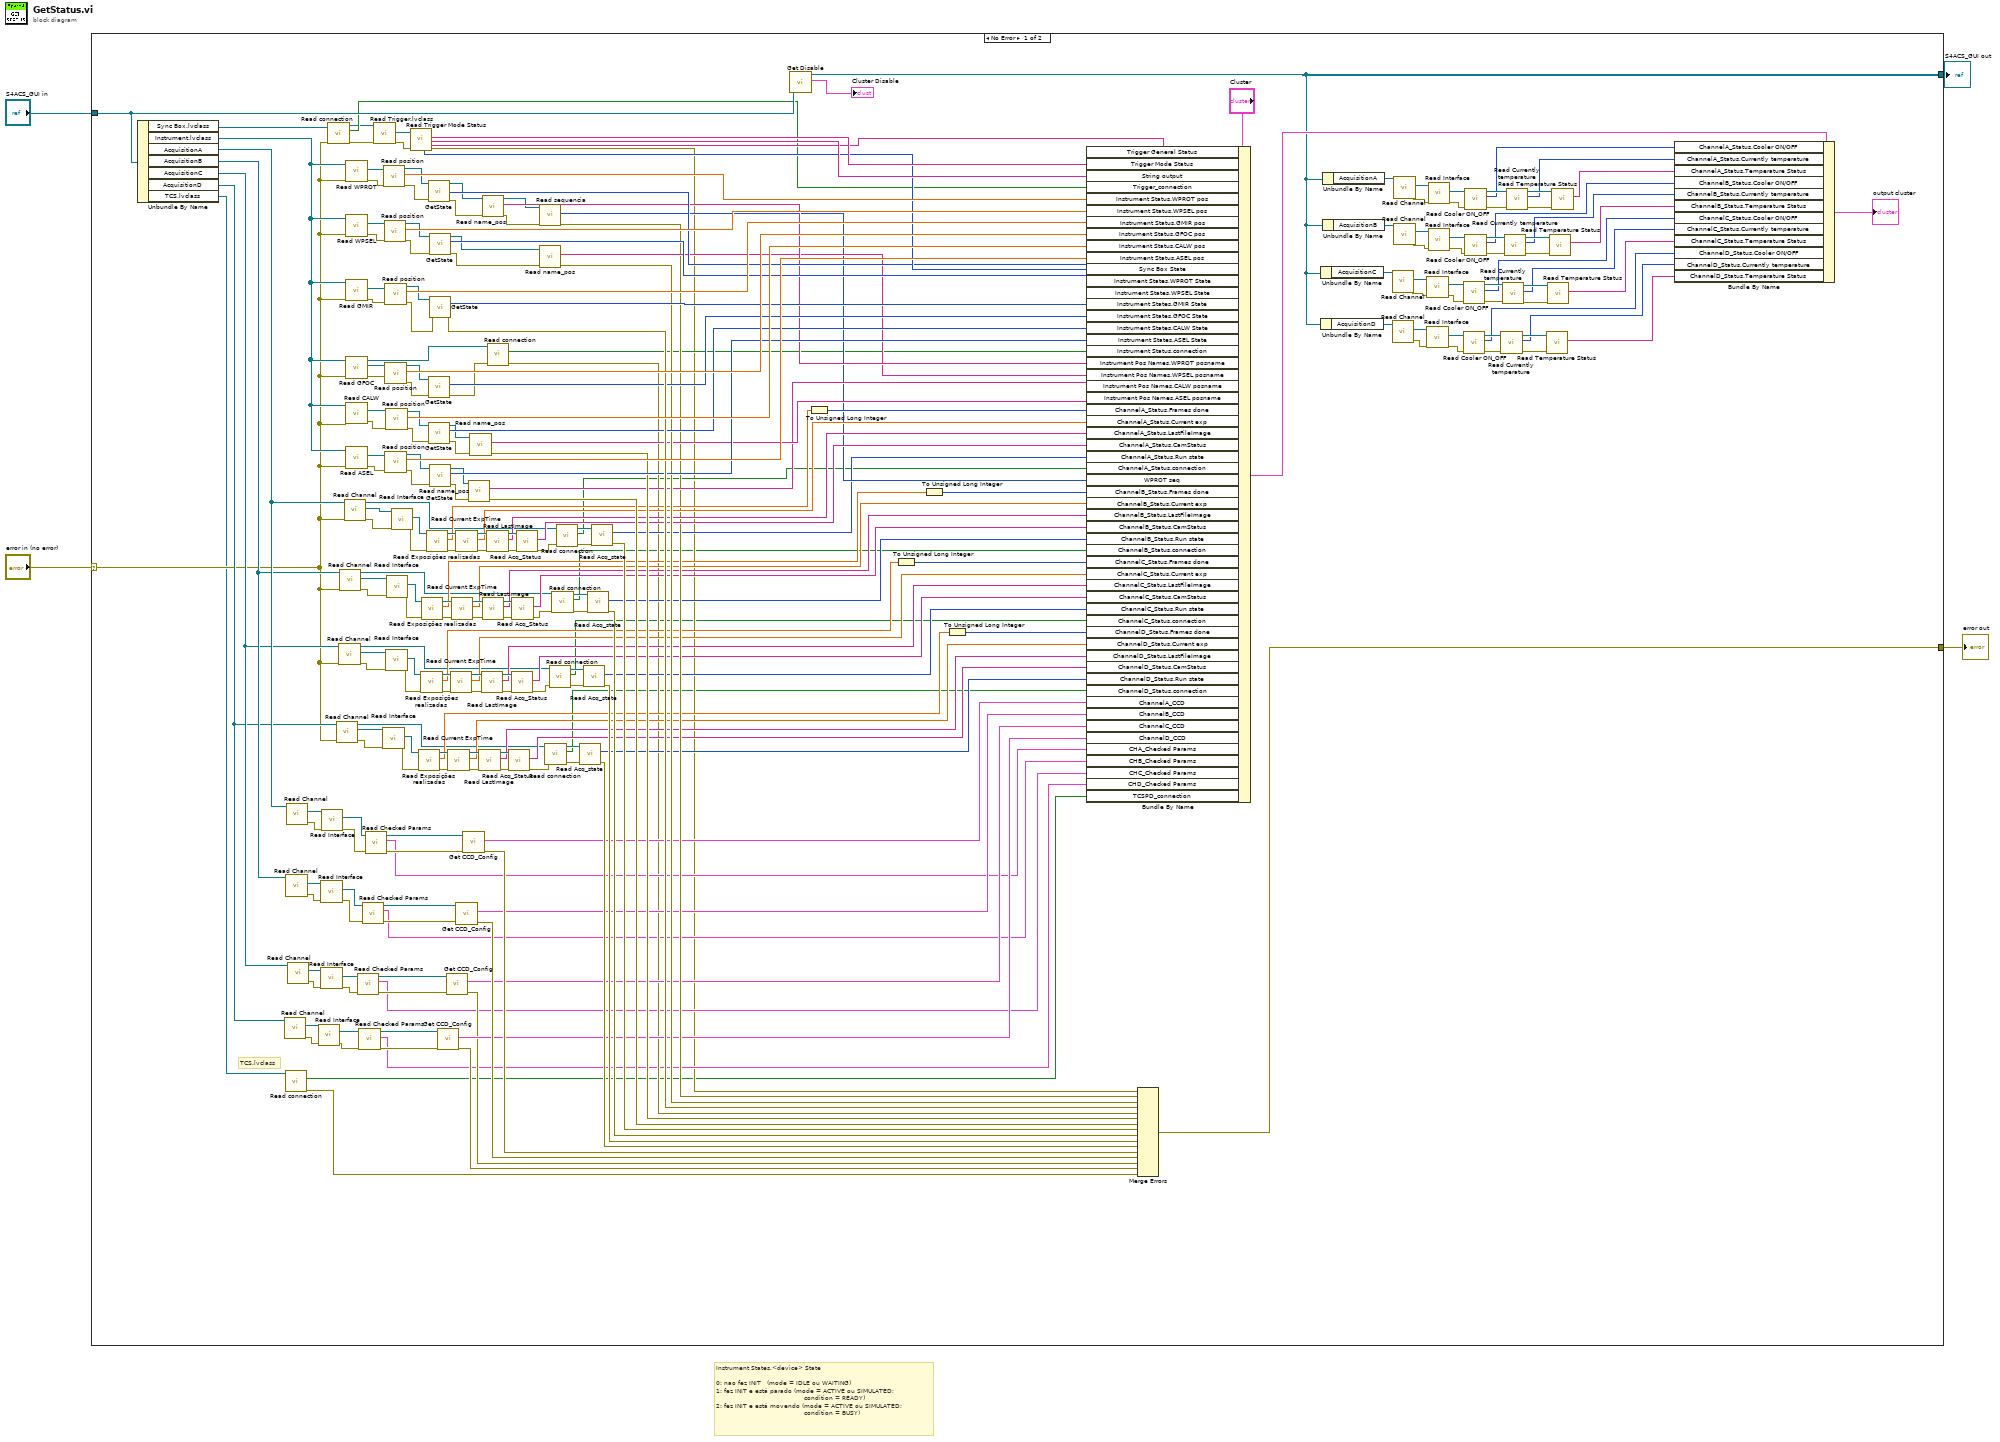
[diagram p0: block diagram]
diagram:
  # "Instrument States.<device> State\n\n0: nao fez INIT   (mode = IDLE ou WAITING)\n1: fez INIT e está parado (mode = ACTIVE ou SIMULATED;\n                                            condition = READY)\n2: fez INIT e está movendo (mode = ACTIVE ou SIMULATED;\n                                            condition = BUSY)"
  n1 = case shown="No Error" "error in (no error)" {
    selector: "error in (no error)" -> [w67 w265]
    tunnel: [w241 w265] -> w3
    tunnel: [w37 w264] -> w1
    tunnel: "S4ACS_GUI in" -> [w166 w264]
    frame No Error {
      # "TCS.lvclass"
      n2 = Unbundle By Name(w166) -> ("Sync Box.lvclass"=w68:refnum<class "Sync Box.lvclass">, "Instrument.lvclass"=w260:refnum<class "Instrument.lvclass">, "AcquisitionA"=w128:refnum<class "Acquisition.lvclass">, "AcquisitionB"=w123:refnum<class "Acquisition.lvclass">, "AcquisitionC"=w118:refnum<class "Acquisition.lvclass">, "AcquisitionD"=w117:refnum<class "Acquisition.lvclass">, "TCS.lvclass"=w58:refnum<class "TCS.lvclass">)
      n3 = call-dynamic "Read Channel.vi"("Acquisition in"=w117) -> ("error out"=w115:errorcluster, "Channel.lvclass"=w116:refnum<class "Channel.lvclass">)  [unwired: 8 in, 1 out]
      n4 = call "Read connection.vi"("Server in"=w58) -> ("error out"=w56:errorcluster, "connection"=w57:bool)  [unwired: 8 in, 1 out]
      n5 = call-dynamic "Read Channel.vi"("Acquisition in"=w123) -> ("error out"=w125:errorcluster, "Channel.lvclass"=w124:refnum<class "Channel.lvclass">)  [unwired: 8 in, 1 out]
      n6 = call-dynamic "Read Channel.vi"("Acquisition in"=w128) -> ("error out"=w129:errorcluster, "Channel.lvclass"=w130:refnum<class "Channel.lvclass">)  [unwired: 8 in, 1 out]
      n7 = call-dynamic "Read Channel.vi"("Acquisition in"=w118) -> ("error out"=w120:errorcluster, "Channel.lvclass"=w119:refnum<class "Channel.lvclass">)  [unwired: 8 in, 1 out]
      n8 = call-dynamic "Read Interface.vi"("error in (no error)"=w115, "Channel in"=w116) -> ("error out"=w97:errorcluster, "Interface.lvclass"=w98:refnum<class "Interface.lvclass">)  [unwired: 7 in, 1 out]
      n9 = call-dynamic "Read Interface.vi"("error in (no error)"=w125, "Channel in"=w124) -> ("error out"=w105:errorcluster, "Interface.lvclass"=w103:refnum<class "Interface.lvclass">)  [unwired: 7 in, 1 out]
      n10 = call-dynamic "Read Interface.vi"("error in (no error)"=w120, "Channel in"=w119) -> ("error out"=w101:errorcluster, "Interface.lvclass"=w99:refnum<class "Interface.lvclass">)  [unwired: 7 in, 1 out]
      n11 = call-dynamic "Read Interface.vi"("error in (no error)"=w129, "Channel in"=w130) -> ("error out"=w110:errorcluster, "Interface.lvclass"=w108:refnum<class "Interface.lvclass">)  [unwired: 7 in, 1 out]
      n12 = call "Read connection.vi"("error in (no error)"=w67, "Server in"=w68) -> ("error out"=w64:errorcluster, "connection"=w69:bool, "Server out"=w66:refnum<class "Sync Box.lvclass">)  [unwired: 7 in]
      n13 = call-dynamic "Read Channel.vi"("error in (no error)"=w67, "Acquisition in"=w117) -> ("error out"=w147:errorcluster, "Channel.lvclass"=w146:refnum<class "Channel.lvclass">, "Acquisition out"=w73:refnum<class "Acquisition.lvclass">)  [unwired: 7 in]
      n14 = call-dynamic "Read Channel.vi"("error in (no error)"=w67, "Acquisition in"=w118) -> ("error out"=w157:errorcluster, "Channel.lvclass"=w156:refnum<class "Channel.lvclass">, "Acquisition out"=w77:refnum<class "Acquisition.lvclass">)  [unwired: 7 in]
      n15 = call-dynamic "Read Channel.vi"("error in (no error)"=w67, "Acquisition in"=w123) -> ("error out"=w175:errorcluster, "Channel.lvclass"=w174:refnum<class "Channel.lvclass">, "Acquisition out"=w81:refnum<class "Acquisition.lvclass">)  [unwired: 7 in]
      n16 = call-dynamic "Read Channel.vi"("error in (no error)"=w67, "Acquisition in"=w128) -> ("error out"=w203:errorcluster, "Channel.lvclass"=w204:refnum<class "Channel.lvclass">, "Acquisition out"=w89:refnum<class "Acquisition.lvclass">)  [unwired: 7 in]
      n17 = call "Read WPROT.vi"("error in (no error)"=w67, "Instrument in"=w260) -> ("error out"=w257:errorcluster, "Opt_Selector.lvclass"=w258:refnum<class "Opt_Selector.lvclass">)  [unwired: 7 in, 1 out]
      n18 = call "Read WPSEL.vi"("error in (no error)"=w67, "Instrument in"=w260) -> ("error out"=w259:errorcluster, "Opt_Selector.lvclass"=w256:refnum<class "Opt_Selector.lvclass">)  [unwired: 7 in, 1 out]
      n19 = call "Read GMIR.vi"("error in (no error)"=w67, "Instrument in"=w260) -> ("error out"=w255:errorcluster, "Opt_Continuous.lvclass"=w253:refnum<class "Opt_Continuous.lvclass">)  [unwired: 7 in, 1 out]
      n20 = call "Read GFOC.vi"("error in (no error)"=w67, "Instrument in"=w260) -> ("error out"=w251:errorcluster, "Opt_Continuous.lvclass"=w252:refnum<class "Opt_Continuous.lvclass">, "Instrument out"=w93:refnum<class "Instrument.lvclass">)  [unwired: 7 in]
      n21 = call "Read CALW.vi"("error in (no error)"=w67, "Instrument in"=w260) -> ("error out"=w254:errorcluster, "Opt_Selector.lvclass"=w250:refnum<class "Opt_Selector.lvclass">)  [unwired: 7 in, 1 out]
      n22 = call "Read ASEL.vi"("error in (no error)"=w67, "Instrument in"=w260) -> ("error out"=w249:errorcluster, "Opt_Selector.lvclass"=w248:refnum<class "Opt_Selector.lvclass">)  [unwired: 7 in, 1 out]
      n23 = call "Read Checked Params.vi"("error in (no error)"=w101, "Interface in"=w99) -> ("error out"=w100:errorcluster, "Checked Params"=w83:T4, "Interface out"=w94:refnum<class "Interface.lvclass">)  [unwired: 7 in]
      n24 = call "Read Checked Params.vi"("error in (no error)"=w97, "Interface in"=w98) -> ("error out"=w96:errorcluster, "Checked Params"=w82:T4, "Interface out"=w95:refnum<class "Interface.lvclass">)  [unwired: 7 in]
      n25 = call "Read Checked Params.vi"("error in (no error)"=w105, "Interface in"=w103) -> ("error out"=w104:errorcluster, "Checked Params"=w84:T4, "Interface out"=w102:refnum<class "Interface.lvclass">)  [unwired: 7 in]
      n26 = call "Read Checked Params.vi"("error in (no error)"=w110, "Interface in"=w108) -> ("error out"=w109:errorcluster, "Checked Params"=w106:T4, "Interface out"=w107:refnum<class "Interface.lvclass">)  [unwired: 7 in]
      n27 = call-dynamic "Read Trigger.lvclass.vi"("error in (no error)"=w64, "Sync Box in"=w66) -> ("error out"=w63:errorcluster, "Trigger.lvclass"=w65:refnum<class "Trigger.lvclass">)  [unwired: 7 in, 1 out]
      n28 = call-dynamic "Read Interface.vi"("error in (no error)"=w147, "Channel in"=w146) -> ("error out"=w152:errorcluster, "Interface.lvclass"=w148:refnum<class "Interface.lvclass">)  [unwired: 7 in, 1 out]
      n29 = call "Read position.vi"("error in (no error)"=w257, "Optics in"=w258) -> ("error out"=w237:errorcluster, "position"=w247:dbl, "Optics out"=w238:refnum<class "Opt_Selector.lvclass">)  [unwired: 7 in]
      n30 = call "Read position.vi"("error in (no error)"=w259, "Optics in"=w256) -> ("error out"=w234:errorcluster, "position"=w246:dbl, "Optics out"=w235:refnum<class "Opt_Selector.lvclass">)  [unwired: 7 in]
      n31 = call "Read position.vi"("error in (no error)"=w255, "Optics in"=w253) -> ("error out"=w231:errorcluster, "position"=w245:dbl, "Optics out"=w232:refnum<class "Opt_Continuous.lvclass">)  [unwired: 7 in]
      n32 = call "Read position.vi"("error in (no error)"=w251, "Optics in"=w252) -> ("error out"=w227:errorcluster, "position"=w244:dbl, "Optics out"=w228:refnum<class "Opt_Continuous.lvclass">)  [unwired: 7 in]
      n33 = call "Read position.vi"("error in (no error)"=w249, "Optics in"=w248) -> ("error out"=w221:errorcluster, "position"=w242:dbl, "Optics out"=w222:refnum<class "Opt_Selector.lvclass">)  [unwired: 7 in]
      n34 = call "Read position.vi"("error in (no error)"=w254, "Optics in"=w250) -> ("error out"=w224:errorcluster, "position"=w243:dbl, "Optics out"=w225:refnum<class "Opt_Selector.lvclass">)  [unwired: 7 in]
      n35 = call-dynamic "Read Interface.vi"("error in (no error)"=w157, "Channel in"=w156) -> ("error out"=w162:errorcluster, "Interface.lvclass"=w158:refnum<class "Interface.lvclass">)  [unwired: 7 in, 1 out]
      n36 = call-dynamic "Read Interface.vi"("error in (no error)"=w175, "Channel in"=w174) -> ("error out"=w180:errorcluster, "Interface.lvclass"=w176:refnum<class "Interface.lvclass">)  [unwired: 7 in, 1 out]
      n37 = call-dynamic "Read Interface.vi"("error in (no error)"=w203, "Channel in"=w204) -> ("error out"=w193:errorcluster, "Interface.lvclass"=w202:refnum<class "Interface.lvclass">)  [unwired: 7 in, 1 out]
      n38 = call-dynamic "Read Trigger Mode Status.vi"("error in (no error)"=w63, "Trigger in"=w65) -> ("error out"=w62:errorcluster, "String output"=w261:string, "Trigger Mode Status"=w262:string, "State"=w240:i32, "Trigger General Status"=w239:string)  [unwired: 4 in, 1 out]
      n39 = call-dynamic "Read Exposições realizadas.vi"("error in (no error)"=w152, "Interface in"=w148) -> ("error out"=w153:errorcluster, "Exposições realizadas"=w138:dbl, "Interface out"=w149:refnum<class "Interface.lvclass">)  [unwired: 7 in]
      n40 = call-dynamic "Read Exposições realizadas.vi"("error in (no error)"=w162, "Interface in"=w158) -> ("error out"=w163:errorcluster, "Exposições realizadas"=w145:dbl, "Interface out"=w159:refnum<class "Interface.lvclass">)  [unwired: 7 in]
      n41 = call-dynamic "Read Exposições realizadas.vi"("error in (no error)"=w180, "Interface in"=w176) -> ("error out"=w181:errorcluster, "Exposições realizadas"=w172:dbl, "Interface out"=w177:refnum<class "Interface.lvclass">)  [unwired: 7 in]
      n42 = call-dynamic "Read Exposições realizadas.vi"("error in (no error)"=w193, "Interface in"=w202) -> ("error out"=w192:errorcluster, "Exposições realizadas"=w197:dbl, "Interface out"=w201:refnum<class "Interface.lvclass">)  [unwired: 7 in]
      n43 = call-dynamic "GetState.vi"("error in (no error)"=w237, "Optics in"=w238) -> ("error out"=w219:errorcluster, "state"=w236:i32, "Optics out"=w218:refnum<class "Opt_Selector.lvclass">)  [unwired: 7 in]
      n44 = call-dynamic "GetState.vi"("error in (no error)"=w227, "Optics in"=w228) -> ("error out"=w92:errorcluster, "state"=w226:i32)  [unwired: 7 in, 1 out]
      n45 = call-dynamic "GetState.vi"("error in (no error)"=w224, "Optics in"=w225) -> ("error out"=w212:errorcluster, "state"=w223:i32, "Optics out"=w210:refnum<class "Opt_Selector.lvclass">)  [unwired: 7 in]
      n46 = call-dynamic "GetState.vi"("error in (no error)"=w234, "Optics in"=w235) -> ("error out"=w215:errorcluster, "state"=w233:i32, "Optics out"=w214:refnum<class "Opt_Selector.lvclass">)  [unwired: 7 in]
      n47 = call-dynamic "GetState.vi"("error in (no error)"=w231, "Optics in"=w232) -> ("error out"=w230:errorcluster, "state"=w229:i32)  [unwired: 7 in, 1 out]
      n48 = call-dynamic "GetState.vi"("error in (no error)"=w221, "Optics in"=w222) -> ("error out"=w208:errorcluster, "state"=w220:i32, "Optics out"=w206:refnum<class "Opt_Selector.lvclass">)  [unwired: 7 in]
      n49 = call-dynamic "Get CCD_Config.vi"("error in (no error)"=w96, "Interface in"=w95) -> ("error out"=w111:errorcluster, "output cluster"=w113:T5)  [unwired: 7 in, 1 out]
      n50 = call-dynamic "Get CCD_Config.vi"("error in (no error)"=w100, "Interface in"=w94) -> ("error out"=w112:errorcluster, "output cluster"=w114:T5)  [unwired: 7 in, 1 out]
      n51 = call-dynamic "Read Current ExpTime.vi"("error in (no error)"=w153, "Interface in"=w149) -> ("error out"=w154:errorcluster, "Current ExpTime"=w136:dbl, "Interface out"=w150:refnum<class "Interface.lvclass">)  [unwired: 7 in]
      n52 = call-dynamic "Read Current ExpTime.vi"("error in (no error)"=w163, "Interface in"=w159) -> ("error out"=w164:errorcluster, "Current ExpTime"=w143:dbl, "Interface out"=w160:refnum<class "Interface.lvclass">)  [unwired: 7 in]
      n53 = call-dynamic "Read Current ExpTime.vi"("error in (no error)"=w181, "Interface in"=w177) -> ("error out"=w182:errorcluster, "Current ExpTime"=w170:dbl, "Interface out"=w178:refnum<class "Interface.lvclass">)  [unwired: 7 in]
      n54 = call-dynamic "Read Current ExpTime.vi"("error in (no error)"=w192, "Interface in"=w201) -> ("error out"=w191:errorcluster, "Current ExpTime"=w198:dbl, "Interface out"=w200:refnum<class "Interface.lvclass">)  [unwired: 7 in]
      n55 = call-dynamic "Get CCD_Config.vi"("error in (no error)"=w104, "Interface in"=w102) -> ("error out"=w122:errorcluster, "output cluster"=w121:T5)  [unwired: 7 in, 1 out]
      n56 = call-dynamic "Get CCD_Config.vi"("error in (no error)"=w109, "Interface in"=w107) -> ("error out"=w126:errorcluster, "output cluster"=w127:T5)  [unwired: 7 in, 1 out]
      n57 = call "Read name_pos.vi"("error in (no error)"=w208, "Optics in"=w206) -> ("error out"=w207:errorcluster, "name_pos"=w205:string)  [unwired: 7 in, 1 out]
      n58 = call "Read name_pos.vi"("error in (no error)"=w212, "Optics in"=w210) -> ("error out"=w211:errorcluster, "name_pos"=w209:string)  [unwired: 7 in, 1 out]
      n59 = call-dynamic "Read LastImage.vi"("error in (no error)"=w154, "Interface in"=w150) -> ("error out"=w155:errorcluster, "LastImage"=w135:string, "Interface out"=w151:refnum<class "Interface.lvclass">)  [unwired: 7 in]
      n60 = call-dynamic "Read LastImage.vi"("error in (no error)"=w164, "Interface in"=w160) -> ("error out"=w165:errorcluster, "LastImage"=w142:string, "Interface out"=w161:refnum<class "Interface.lvclass">)  [unwired: 7 in]
      n61 = call "Read name_pos.vi"("error in (no error)"=w219, "Optics in"=w218) -> ("error out"=w188:errorcluster, "name_pos"=w217:string, "Optics out"=w189:refnum<class "Opt_Selector.lvclass">)  [unwired: 7 in]
      n62 = call-dynamic "Read LastImage.vi"("error in (no error)"=w182, "Interface in"=w178) -> ("error out"=w183:errorcluster, "LastImage"=w169:string, "Interface out"=w179:refnum<class "Interface.lvclass">)  [unwired: 7 in]
      n63 = call-dynamic "Read LastImage.vi"("error in (no error)"=w191, "Interface in"=w200) -> ("error out"=w190:errorcluster, "LastImage"=w195:string, "Interface out"=w199:refnum<class "Interface.lvclass">)  [unwired: 7 in]
      n64 = call "Read connection.vi"("error in (no error)"=w92, "Server in"=w93) -> ("error out"=w91:errorcluster, "connection"=w90:bool)  [unwired: 7 in, 1 out]
      n65 = call-dynamic "Read Acq_Status.vi"("error in (no error)"=w155, "Interface in"=w151) -> ("error out"=w72:errorcluster, "Acq_Status"=w134:string)  [unwired: 7 in, 1 out]
      n66 = call-dynamic "Read Acq_Status.vi"("error in (no error)"=w165, "Interface in"=w161) -> ("error out"=w75:errorcluster, "Acq_Status"=w141:string)  [unwired: 7 in, 1 out]
      n67 = call-dynamic "Read Acq_Status.vi"("error in (no error)"=w183, "Interface in"=w179) -> ("error out"=w79:errorcluster, "Acq_Status"=w168:string)  [unwired: 7 in, 1 out]
      n68 = call-dynamic "Read Acq_Status.vi"("error in (no error)"=w190, "Interface in"=w199) -> ("error out"=w87:errorcluster, "Acq_Status"=w194:string)  [unwired: 7 in, 1 out]
      n69 = call-dynamic "Read sequencia.vi"("error in (no error)"=w188, "Opt_Selector in"=w189) -> ("error out"=w187:errorcluster, "sequencia"=w186:u16)  [unwired: 7 in, 1 out]
      n70 = call "Read name_pos.vi"("error in (no error)"=w215, "Optics in"=w214) -> ("error out"=w216:errorcluster, "name_pos"=w213:string)  [unwired: 7 in, 1 out]
      n71 = call "Read connection.vi"("error in (no error)"=w72, "Server in"=w73) -> ("error out"=w71:errorcluster, "connection"=w59:bool, "Server out"=w70:refnum<class "Acquisition.lvclass">)  [unwired: 7 in]
      n72 = call "Read connection.vi"("error in (no error)"=w75, "Server in"=w77) -> ("error out"=w74:errorcluster, "connection"=w60:bool, "Server out"=w76:refnum<class "Acquisition.lvclass">)  [unwired: 7 in]
      n73 = call "Read connection.vi"("error in (no error)"=w79, "Server in"=w81) -> ("error out"=w78:errorcluster, "connection"=w61:bool, "Server out"=w80:refnum<class "Acquisition.lvclass">)  [unwired: 7 in]
      n74 = call "Read connection.vi"("error in (no error)"=w87, "Server in"=w89) -> ("error out"=w86:errorcluster, "connection"=w85:bool, "Server out"=w88:refnum<class "Acquisition.lvclass">)  [unwired: 7 in]
      n75 = call-dynamic "Read Acq_state.vi"("error in (no error)"=w71, "Acquisition in"=w70) -> ("error out"=w132:errorcluster, "Acq_state"=w133:u32)  [unwired: 7 in, 1 out]
      n76 = call-dynamic "Read Acq_state.vi"("error in (no error)"=w74, "Acquisition in"=w76) -> ("error out"=w139:errorcluster, "Acq_state"=w140:u32)  [unwired: 7 in, 1 out]
      n77 = call-dynamic "Read Acq_state.vi"("error in (no error)"=w78, "Acquisition in"=w80) -> ("error out"=w173:errorcluster, "Acq_state"=w167:u32)  [unwired: 7 in, 1 out]
      n78 = call-dynamic "Read Acq_state.vi"("error in (no error)"=w86, "Acquisition in"=w88) -> ("error out"=w184:errorcluster, "Acq_state"=w185:u32)  [unwired: 7 in, 1 out]
      n79 = call-dynamic "Get Disable.vi"("S4ACS_GUI in"=w166) -> ("Cluster Disable"=→"Cluster Disable":T1, "S4ACS_GUI out"=w37:refnum<class "S4GUI.lvclass">)  [unwired: 8 in, 1 out]
      n80 = To Unsigned Long Integer(number=w197) -> (unsigned 32bit integer=w196:u32)
      n81 = To Unsigned Long Integer(number=w145) -> (unsigned 32bit integer=w144:u32)
      n82 = To Unsigned Long Integer(number=w172) -> (unsigned 32bit integer=w171:u32)
      n83 = To Unsigned Long Integer(number=w138) -> (unsigned 32bit integer=w137:u32)
      n84 = Bundle By Name(cluster="Cluster", "Trigger General Status"=w239, "Trigger Mode Status"=w262, "String output"=w261, "Trigger_connection"=w69, "Instrument Status.WPROT pos"=w247, "Instrument Status.WPSEL pos"=w246, "Instrument Status.GMIR pos"=w245, "Instrument Status.GFOC pos"=w244, "Instrument Status.CALW pos"=w243, "Instrument Status.ASEL pos"=w242, "Sync Box State"=w240, "Instrument States.WPROT State"=w236, "Instrument States.WPSEL State"=w233, "Instrument States.GMIR State"=w229, "Instrument States.GFOC State"=w226, "Instrument States.CALW State"=w223, "Instrument States.ASEL State"=w220, "Instrument Status.connection"=w90, "Instrument Pos Names.WPROT posname"=w217, "Instrument Pos Names.WPSEL posname"=w213, "Instrument Pos Names.CALW posname"=w209, "Instrument Pos Names.ASEL posname"=w205, "ChannelA_Status.Frames done"=w196, "ChannelA_Status.Current exp"=w198, "ChannelA_Status.LastFileImage"=w195, "ChannelA_Status.CamStatus"=w194, "ChannelA_Status.Run state"=w185, "ChannelA_Status.connection"=w85, "WPROT seq"=w186, "ChannelB_Status.Frames done"=w171, "ChannelB_Status.Current exp"=w170, "ChannelB_Status.LastFileImage"=w169, "ChannelB_Status.CamStatus"=w168, "ChannelB_Status.Run state"=w167, "ChannelB_Status.connection"=w61, "ChannelC_Status.Frames done"=w144, "ChannelC_Status.Current exp"=w143, "ChannelC_Status.LastFileImage"=w142, "ChannelC_Status.CamStatus"=w141, "ChannelC_Status.Run state"=w140, "ChannelC_Status.connection"=w60, "ChannelD_Status.Frames done"=w137, "ChannelD_Status.Current exp"=w136, "ChannelD_Status.LastFileImage"=w135, "ChannelD_Status.CamStatus"=w134, "ChannelD_Status.Run state"=w133, "ChannelD_Status.connection"=w59, "ChannelA_CCD"=w127, "ChannelB_CCD"=w121, "ChannelC_CCD"=w114, "ChannelD_CCD"=w113, "CHA_Checked Params"=w106, "CHB_Checked Params"=w84, "CHC_Checked Params"=w83, "CHD_Checked Params"=w82, "TCSPD_connection"=w57) -> (w55:T3)
      n85 = Merge Errors(w62, w187, w216, w230, w91, w211, w207, w184, w173, w139, w132, w126, w122, w112, w111, w56) -> (w241:errorcluster)
      n86 = Unbundle By Name(w37) -> ("AcquisitionC"=w42:refnum<class "Acquisition.lvclass">)
      n87 = Unbundle By Name(w37) -> ("AcquisitionD"=w38:refnum<class "Acquisition.lvclass">)
      n88 = Unbundle By Name(w37) -> ("AcquisitionA"=w50:refnum<class "Acquisition.lvclass">)
      n89 = Unbundle By Name(w37) -> ("AcquisitionB"=w46:refnum<class "Acquisition.lvclass">)
      n90 = call-dynamic "Read Channel.vi"("Acquisition in"=w42) -> ("error out"=w44:errorcluster, "Channel.lvclass"=w45:refnum<class "Channel.lvclass">)  [unwired: 8 in, 1 out]
      n91 = call-dynamic "Read Channel.vi"("Acquisition in"=w38) -> ("error out"=w40:errorcluster, "Channel.lvclass"=w41:refnum<class "Channel.lvclass">)  [unwired: 8 in, 1 out]
      n92 = call-dynamic "Read Channel.vi"("Acquisition in"=w50) -> ("error out"=w53:errorcluster, "Channel.lvclass"=w54:refnum<class "Channel.lvclass">)  [unwired: 8 in, 1 out]
      n93 = call-dynamic "Read Channel.vi"("Acquisition in"=w46) -> ("error out"=w48:errorcluster, "Channel.lvclass"=w49:refnum<class "Channel.lvclass">)  [unwired: 8 in, 1 out]
      n94 = call-dynamic "Read Interface.vi"("error in (no error)"=w44, "Channel in"=w45) -> ("error out"=w15:errorcluster, "Interface.lvclass"=w43:refnum<class "Interface.lvclass">)  [unwired: 7 in, 1 out]
      n95 = call-dynamic "Read Interface.vi"("error in (no error)"=w40, "Channel in"=w41) -> ("error out"=w14:errorcluster, "Interface.lvclass"=w39:refnum<class "Interface.lvclass">)  [unwired: 7 in, 1 out]
      n96 = call-dynamic "Read Interface.vi"("error in (no error)"=w53, "Channel in"=w54) -> ("error out"=w31:errorcluster, "Interface.lvclass"=w52:refnum<class "Interface.lvclass">)  [unwired: 7 in, 1 out]
      n97 = call-dynamic "Read Interface.vi"("error in (no error)"=w48, "Channel in"=w49) -> ("error out"=w25:errorcluster, "Interface.lvclass"=w47:refnum<class "Interface.lvclass">)  [unwired: 7 in, 1 out]
      n98 = call-dynamic "Read Cooler ON_OFF.vi"("error in (no error)"=w15, "Interface in"=w43) -> ("error out"=w16:errorcluster, "Cooler ON/OFF"=w10:i16, "Interface out"=w18:refnum<class "Interface.lvclass">)  [unwired: 7 in]
      n99 = call-dynamic "Read Cooler ON_OFF.vi"("error in (no error)"=w14, "Interface in"=w39) -> ("error out"=w13:errorcluster, "Cooler ON/OFF"=w7:i16, "Interface out"=w12:refnum<class "Interface.lvclass">)  [unwired: 7 in]
      n100 = call-dynamic "Read Cooler ON_OFF.vi"("error in (no error)"=w31, "Interface in"=w52) -> ("error out"=w30:errorcluster, "Cooler ON/OFF"=w34:i16, "Interface out"=w36:refnum<class "Interface.lvclass">)  [unwired: 7 in]
      n101 = call-dynamic "Read Cooler ON_OFF.vi"("error in (no error)"=w25, "Interface in"=w47) -> ("error out"=w26:errorcluster, "Cooler ON/OFF"=w23:i16, "Interface out"=w24:refnum<class "Interface.lvclass">)  [unwired: 7 in]
      n102 = call-dynamic "Read Currently temperature.vi"("error in (no error)"=w13, "Interface in"=w12) -> ("error out"=w19:errorcluster, "Currently temperature"=w6:i8, "Interface out"=w11:refnum<class "Interface.lvclass">)  [unwired: 7 in]
      n103 = call-dynamic "Read Currently temperature.vi"("error in (no error)"=w16, "Interface in"=w18) -> ("error out"=w20:errorcluster, "Currently temperature"=w9:i8, "Interface out"=w17:refnum<class "Interface.lvclass">)  [unwired: 7 in]
      n104 = call-dynamic "Read Currently temperature.vi"("error in (no error)"=w26, "Interface in"=w24) -> ("error out"=w27:errorcluster, "Currently temperature"=w22:i8, "Interface out"=w28:refnum<class "Interface.lvclass">)  [unwired: 7 in]
      n105 = call-dynamic "Read Currently temperature.vi"("error in (no error)"=w30, "Interface in"=w36) -> ("error out"=w29:errorcluster, "Currently temperature"=w33:i8, "Interface out"=w35:refnum<class "Interface.lvclass">)  [unwired: 7 in]
      n106 = call-dynamic "Read Temperature Status.vi"("error in (no error)"=w19, "Interface in"=w11) -> ("Temperature Status"=w5:string)  [unwired: 7 in, 2 out]
      n107 = call-dynamic "Read Temperature Status.vi"("error in (no error)"=w20, "Interface in"=w17) -> ("Temperature Status"=w8:string)  [unwired: 7 in, 2 out]
      n108 = call-dynamic "Read Temperature Status.vi"("error in (no error)"=w27, "Interface in"=w28) -> ("Temperature Status"=w21:string)  [unwired: 7 in, 2 out]
      n109 = call-dynamic "Read Temperature Status.vi"("error in (no error)"=w29, "Interface in"=w35) -> ("Temperature Status"=w32:string)  [unwired: 7 in, 2 out]
      n110 = Bundle By Name(cluster=w55, "ChannelA_Status.Cooler ON/OFF"=w34, "ChannelA_Status.Currently temperature"=w33, "ChannelA_Status.Temperature Status"=w32, "ChannelB_Status.Cooler ON/OFF"=w23, "ChannelB_Status.Currently temperature"=w22, "ChannelB_Status.Temperature Status"=w21, "ChannelC_Status.Cooler ON/OFF"=w10, "ChannelC_Status.Currently temperature"=w9, "ChannelC_Status.Temperature Status"=w8, "ChannelD_Status.Cooler ON/OFF"=w7, "ChannelD_Status.Currently temperature"=w6, "ChannelD_Status.Temperature Status"=w5) -> (→"output cluster":T3)
    }
    frame Error {
    }
  }
  "error out" <- w3
  "S4ACS_GUI out" <- w1
